vi "TLB Native Dynamic Events ver 0.17c.vi"() -> ()   [LabVIEW 2018]
uses:
  Labview Training Phase 2/Enum Controls/States for Action Engine.ctl
  TLB Type Definitions/State Type Definitions, for 0.26d versions and later.ctl
  TLB Type Definitions/Intruction Type Definitions.ctl
  TLB Type Definitions/Encoder cluster.ctl
  TLB Type Definitions/PING CLUSTER.ctl
  <vilib>/Studica/Studica Toolkit/NavX/NavX.lvlib
  <vilib>/Studica/Studica Toolkit/Background/DIO Channel.ctl
  Underlying VI's/NavX VI/navX type def.ctl
  <vilib>/Studica/Studica Toolkit/Background/I2C Channel.ctl
  TLB Type Definitions/Vision cluster.ctl
  <vilib>/NI_Real-Time Target Support.lvlib
  TLB Type Definitions/Stepper cluster.ctl
  Experimental VI's/Archived VI's/MOTOR CONTROL NO PID Type Def.ctl
  Underlying VI's/I2C Master VI/I2C MASTER Type Def.ctl
  Underlying VI's/I2C Master VI/I2C_MASTER_WRITE_NEW Type Def.ctl
  <vilib>/userdefined/High Color/IMAQdx.ctl
  Underlying VI's/I2C Master VI/Arduino_Interfacing.ctl
  TLB Type Definitions/Yaw Cluster.ctl
  TLB Type Definitions/Time cluster.ctl
  TLB Type Definitions/Y Stepper cluster.ctl
  Underlying VI's/Modified webcam FGV/Webcam AE.ctl
  Underlying VI's/Elasped Timer/Elapsed timer control.ctl
  Underlying VI's/Motor Control VI with PID/MOTOR CONTROL WITH PID AE DATA MODE TYPE DEF.ctl
  Underlying VI's/Motor Control VI with PID/MOTOR CONTROL WITH PID AE DIRECTION TYPE DEF.ctl
  TLB Type Definitions/IR Sensor Type Def.ctl
  <vilib>/myRIO/Common/Instrument Driver Framework/myRIO v1.0/AI/typedefs/AI Channels Enum.ctl
  <vilib>/myRIO/Common/Instrument Driver Framework/myRIO v1.0/AI/typedefs/AI Channels List.ctl
  <vilib>/Utility/RT CPU Load.ctl
panel:
  out "Left IR Sensor":dbl
  out "Obstacle detected":bool
  out "Speed & distance":T1
  out "Object Center Coordinates":cluster{"x":sgl, "y":sgl}
  out "Object detection cluster":T2
  out "Time up flag":bool
  out "Task selection":u8
  in  "Object recognition mode":enum16{"Ball", "Soap", "Gel", "Pipe", "None"}(ring)
  out "NavX Readings":T3
  out "Arduino Data":T4
  out "CPU loads":T5[](array[typedef]) {"ISR (%)" format="%#.2f"; "Idle (%)" format="%#.2f"; "Background (%)" format="%#.2f"; "Normal (%)" format="%#.2f"; "Above Normal (%)" format="%#.2f"; "High (%)" format="%#.2g"; "Timed Structures (%)" format="%#.2g"; "Time Critical (%)" format="%#.2g"; "Total (%)" format="%#.2g"}
  out "TASK ENABLE":bool
  out "Rising Edge":bool
  in  "Green LED":bool
  out "I2C Error":errorcluster
  out "State Logic":T6=enum."Startup"
  out "elements":T7[](array[typedef])
  in  "STOP TASK":bool
  in  "OK Button":bool
  in  "STOP":bool
  out "error out":errorcluster
  out "Action Queue Items":i32
  out "State Logic Queue Items":i32
  out "Action Queues items":string[](array[string])=["Hardware reset", "Software reset", ""]
  out "Action State":string
  # "System Health Status Update"
  # "VISION"
  # "TLB FRAMEWORK STATUS"
  # "Test Programme written by Calvin Loke    Dated: 28 Aug 2019\nTest Programme revised by Dr Alex See   Dated 30 Aug 2019\n\nRevision date: 20/03/2020\nProgramme version:   TLB Native Dynamic Events ver 0.14a"
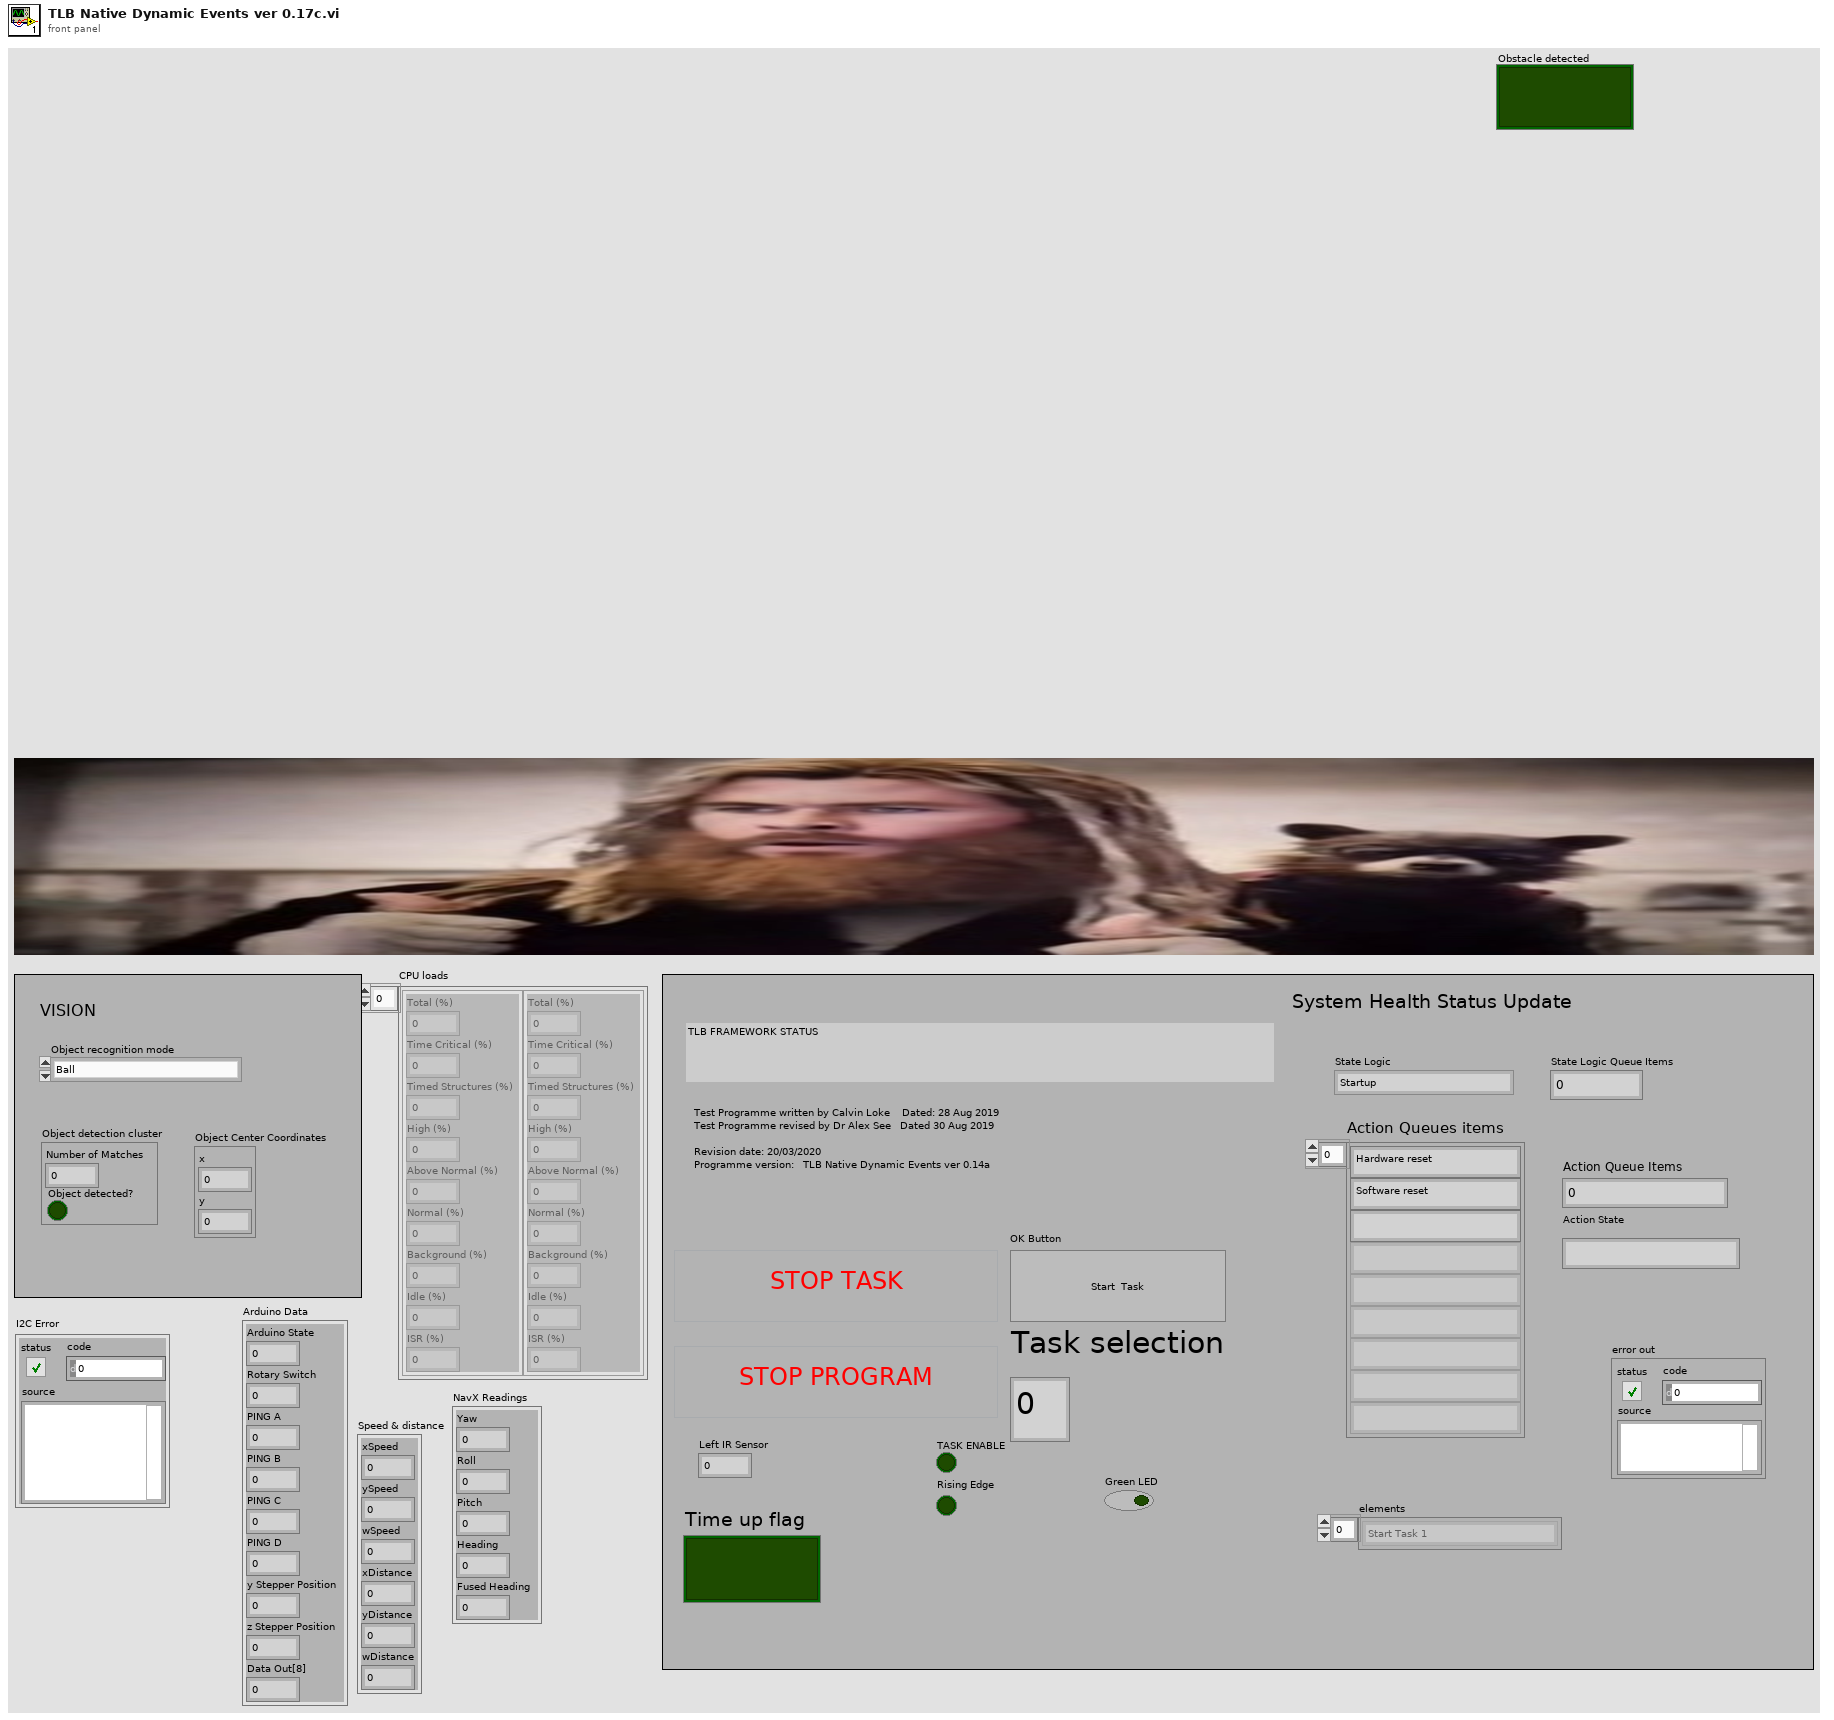
[diagram p1: front panel]
types:
  T1 = cluster{"xSpeed":dbl, "ySpeed":dbl, "wSpeed":dbl, "xDistance":dbl, "yDistance":dbl, "wDistance":dbl}
  T2 = cluster{"Number of Matches":i32, "Object detected?":bool}
  T3 = cluster{"Yaw":dbl, "Roll":dbl, "Pitch":dbl, "Heading":dbl, "Fused Heading":dbl}
  T4 = cluster{"Arduino State":u8, "Rotary Switch":u8, "PING A":u8, "PING B":u8, "PING C":u8, "PING D":u8, "y Stepper Position":u8, "z Stepper Position":u8, "Data Out[8]":u8}
  T5 = typedef "NI_Real-Time Target Support.lvlib/RT CPU Load.ctl" = cluster{"Total (%)":dbl, "Time Critical (%)":dbl, "Timed Structures (%)":dbl, "High (%)":dbl, "Above Normal (%)":dbl, "Normal (%)":dbl, "Background (%)":dbl, "Idle (%)":dbl, "ISR (%)":dbl}
  T6 = typedef "State Type Definitions.ctl" = enum16{"None", "Startup", "Move to Angle", "True Stop", "Idle", "Shutdown", "Task 1A", "Task 1B", "Task 2:Raise Arm", "Task 2:Sensor Mode", "Task 2:Reverse Mode", "Task 3", "Task 4_A", "Task 4_B", "Task 4_C", "Task 4_D", "Task 5A", "Task 5B", "Task 5C", "Task 5D", "Task 5E: POSITION ARM", "Task 5F: ARM GRAB HEIGHT", "Task 5G: CLOSE CLAW", "Task 5H: RAISE ARM", "Task 6_A", "Task 6_B", "Task 7", "Task 8A: RAISE ARM", "Task 8B: MOVE TO BOX", "Task 8C: CAM BURST", "Task 8D: PROCESS IMAGE", "Task 8E: ROBOT ADJUST", "Task 8F: CAM BURST 2", "Task 8G: PROCESS IMAGE 2", "Task 8H: ARM ADJUST", "Task 8I: ARM GRAB HEIGHT", "Task 8J: CLOSE CLAW", "Task 8K: RAISE MY SWORD", "Task 9A: Raise Arm", "Task 9B: Rotate to Angle", "Task 9C: Detect Box", "Task 9D: MOVE FORWARD", "Task 9E: MOVE LEFT", "Task 9F: SCAN IMAGE", "Task 9G: PROCESS COLOUR", "Task 9H: MOVE RIGHT", "Task 9I: SCAN IMAGE", "Task 9J: PROCESS COLOUR", "Task 9K: ROTATE 90 CW", "Task 9L: MOVE FORWARD", "Task 9M: MOVE RIGHT", "Task 9N: SCAN IMAGE", "Task 9O: PROCESS COLOUR", "Task 9P: MOVE RIGHT", "Task 9Q: SCAN IMAGE", "Task 9R: PROCESS COLOUR", "Task A1: Raise Arm", "Task A2: Rotate to Angle", "Task A3: Move Forward", "Task A4: Rotate CW 90"}
  T7 = typedef "Intruction Type Definitions.ctl" = enum16{"None", "Start Task 1", "Start Task 2", "Start Task 3", "Start Task 4", "Start Task 5", "Start Task 6", "Start Task 7", "Start Task 8 - BALL", "Start Task 8 - Gel", "Start Task 8 - Pipe", "Start Task 8 - Soap", "Start Task 9", "Start Task A", "Start Task B", "Exit"}
  T8 = typedef "IR Sensor Type Def.ctl" = cluster{"Left IR Sensor":dbl, "Arm IR Sensor":dbl, "Bottom IR Sensor":dbl}
  T9 = typedef "Y Stepper cluster.ctl" = cluster{"yStepper desired":u8}
  T10 = typedef "Time cluster.ctl" = cluster{"Time up flag":bool, "SET TIME TO CHECK":dbl}
  T11 = typedef "Yaw Cluster.ctl" = cluster{"Yaw":dbl, "Compass":dbl}
  T12 = typedef "Stepper cluster.ctl" = cluster{"y Stepper Position":u8, "z Stepper Position":u8}
  T13 = typedef "DIO Channel.ctl" = enum16{"Not Connected", "A/DIO1", "A/DIO2", "A/DIO3", "A/DIO4", "A/DIO5", "A/DIO6", "A/DIO7", "A/DIO13", "B/DIO1", "B/DIO2", "B/DIO3", "B/DIO4", "B/DIO5", "B/DIO6", "B/DIO7", "B/DIO13", "C/DIO0", "C/DIO1", "C/DIO2", "C/DIO3", "C/DIO4", "C/DIO5", "C/DIO6", "C/DIO7"}
  T14 = typedef "Vision cluster.ctl" = cluster{"Recognized Object":bool, "Object X coordinate":dbl, "Object Y coordinate":dbl}
  T15 = typedef "PING CLUSTER.ctl" = cluster{"PING_A":u8, "PING_B":u8, "PING_C":u8, "PING_D":u8}
  T16 = typedef "Encoder cluster.ctl" = cluster{"xDistance":dbl, "yDistance":dbl, "wDistance":dbl}
  T17 = cluster{"DIO Channel":T13, "FPGA VI Reference Out":refnum<k20>}
  T18 = typedef "navX type def.ctl" = enum16{"Get i2C reference", "Read Values", "Zero Yaw"}
  T19 = typedef "Arduino_Interfacing.ctl" = enum16{"Initialize", "Write to Arduino", "Read From Arduino"}
  T20 = typedef "I2C Channel.ctl" = enum16{"Not Connected", "A", "B"}
  T21 = typedef "States for Action Engine.ctl" = enum16{"Initialize", "Write", "Read"}
  T22 = cluster{"I2C Ref Out":cluster{"I2C Channel":T20, "FPGA VI Reference Out":refnum<k20>}, "Connected":bool, "Slave Address (7-bit)":u8, "Registry":u8[]}
  T23 = typedef "IMAQ Image.ctl" = refnum<image>
  T24 = typedef "State Type Definitions.ctl" = enum16{"None", "Startup", "Move to Angle", "True Stop", "Idle", "Shutdown", "Task 1", "Task 2:Raise Arm", "Task 2:Sensor Mode", "Task 2:Reverse Mode", "Task 3", "Task 4_A", "Task 4_B", "Task 4_C", "Task 4_D", "Task 5A: ARM CAM HEIGHT", "Task 5B: MOVE TO BOX", "Task 5C: CAM BURST", "Task 5D: PROCESS IMAGE", "Task 5E: POSITION ARM", "Task 5F: ARM GRAB HEIGHT", "Task 5G: CLOSE CLAW", "Task 5H: RAISE ARM", "Task 5_F", "Task 5G", "Task 5H", "Task 5I", "Task 6_A", "Task 6_B", "Task 7", "Task 8", "Task 9A: Raise Arm", "Task 9B: Rotate to Angle", "Task 9C: Rotation alignmnet", "Task B"}
  T25 = typedef "MOTOR CONTROL WITH PID AE DIRECTION TYPE DEF.ctl" = enum16{"y-axis movement", "x-axis movement", "rotation", "stop", "reset encoders"}
  T26 = typedef "MOTOR CONTROL WITH PID AE DATA MODE TYPE DEF.ctl" = enum16{"Init AE", "Write to AE", "Read from AE"}
  T27 = typedef "Elapsed timer control.ctl" = enum16{"Start", "Pause", "Initialize"}
  T28 = typedef "I2C_MASTER_WRITE_NEW Type Def.ctl" = enum16{"Ultrasonic sensors", "Stepper origin", "zStepper 13.3k", "zStepper 13k", "zStepper 12k", "zStepper 11k", "zStepper 10k", "zStepper 9k", "zStepper 8k", "zStepper 7k", "zStepper 6k", "zStepper 5k", "zStepper 4k", "zStepper 3k", "zStepper 2k", "zStepper 1k", "zStepper 900", "zStepper 800", "zStepper 700", "zStepper 600", "zStepper 500", "zStepper 400", "zStepper 300", "zStepper 200", "zStepper 100", "zStepper 0", "yStepper control", "Open Claw", "Close Claw", "Soft Reset"}
  T29 = typedef "Webcam AE.ctl" = enum16{"Initialize Camera", "Open Camera", "Continuous Acquisition", "Close Camera", "Retrieve Image", "Dispose Camera Image Buffer"}
  T30 = typedef "IMAQdx.ctl" = refnum<k21>
  T31 = typedef "Webcam AE.ctl" = enum16{"Initialize Camera", "Open Camera", "Continuous Acquisition", "Close Camera", "Retrieve Image", "Dispose Image Buffers"}
  T32 = typedef "MOTOR CONTROL NO PID Type Def.ctl" = enum16{"Init", "Front Back", "Left Right", "Rotate", "Stop", "Latch"}
  T33 = typedef "AI Channels List.ctl" = T34[]
  T34 = typedef "AI Channels Enum.ctl" = enum16{"Not Connected", "AudioIn/Left", "AudioIn/Right", "C/AI0", "C/AI1", "A/AI0", "A/AI1", "A/AI2", "A/AI3", "A/AI4", "A/AI5", "A/AI6", "A/AI7", "B/AI0", "B/AI1", "B/AI2", "B/AI3", "B/AI4", "B/AI5", "B/AI6", "B/AI7", "AI/AI0", "AI/AI1", "AI/AI2", "AI/AI3", "A/AI0 (DIFF)", "A/AI1 (DIFF)", "A/AI2 (DIFF)", "A/AI3 (DIFF)", "B/AI0 (DIFF)", "B/AI1 (DIFF)", "B/AI2 (DIFF)", "B/AI3 (DIFF)"}
  T35 = typedef "I2C MASTER Type Def.ctl" = enum16{"Last State", "Mode 0", "Mode 1", "Mode 2", "Mode 3", "Mode 4", "Mode 5", "Mode 6", "Mode 7", "Mode 8", "Mode 9", "Mode 10"}
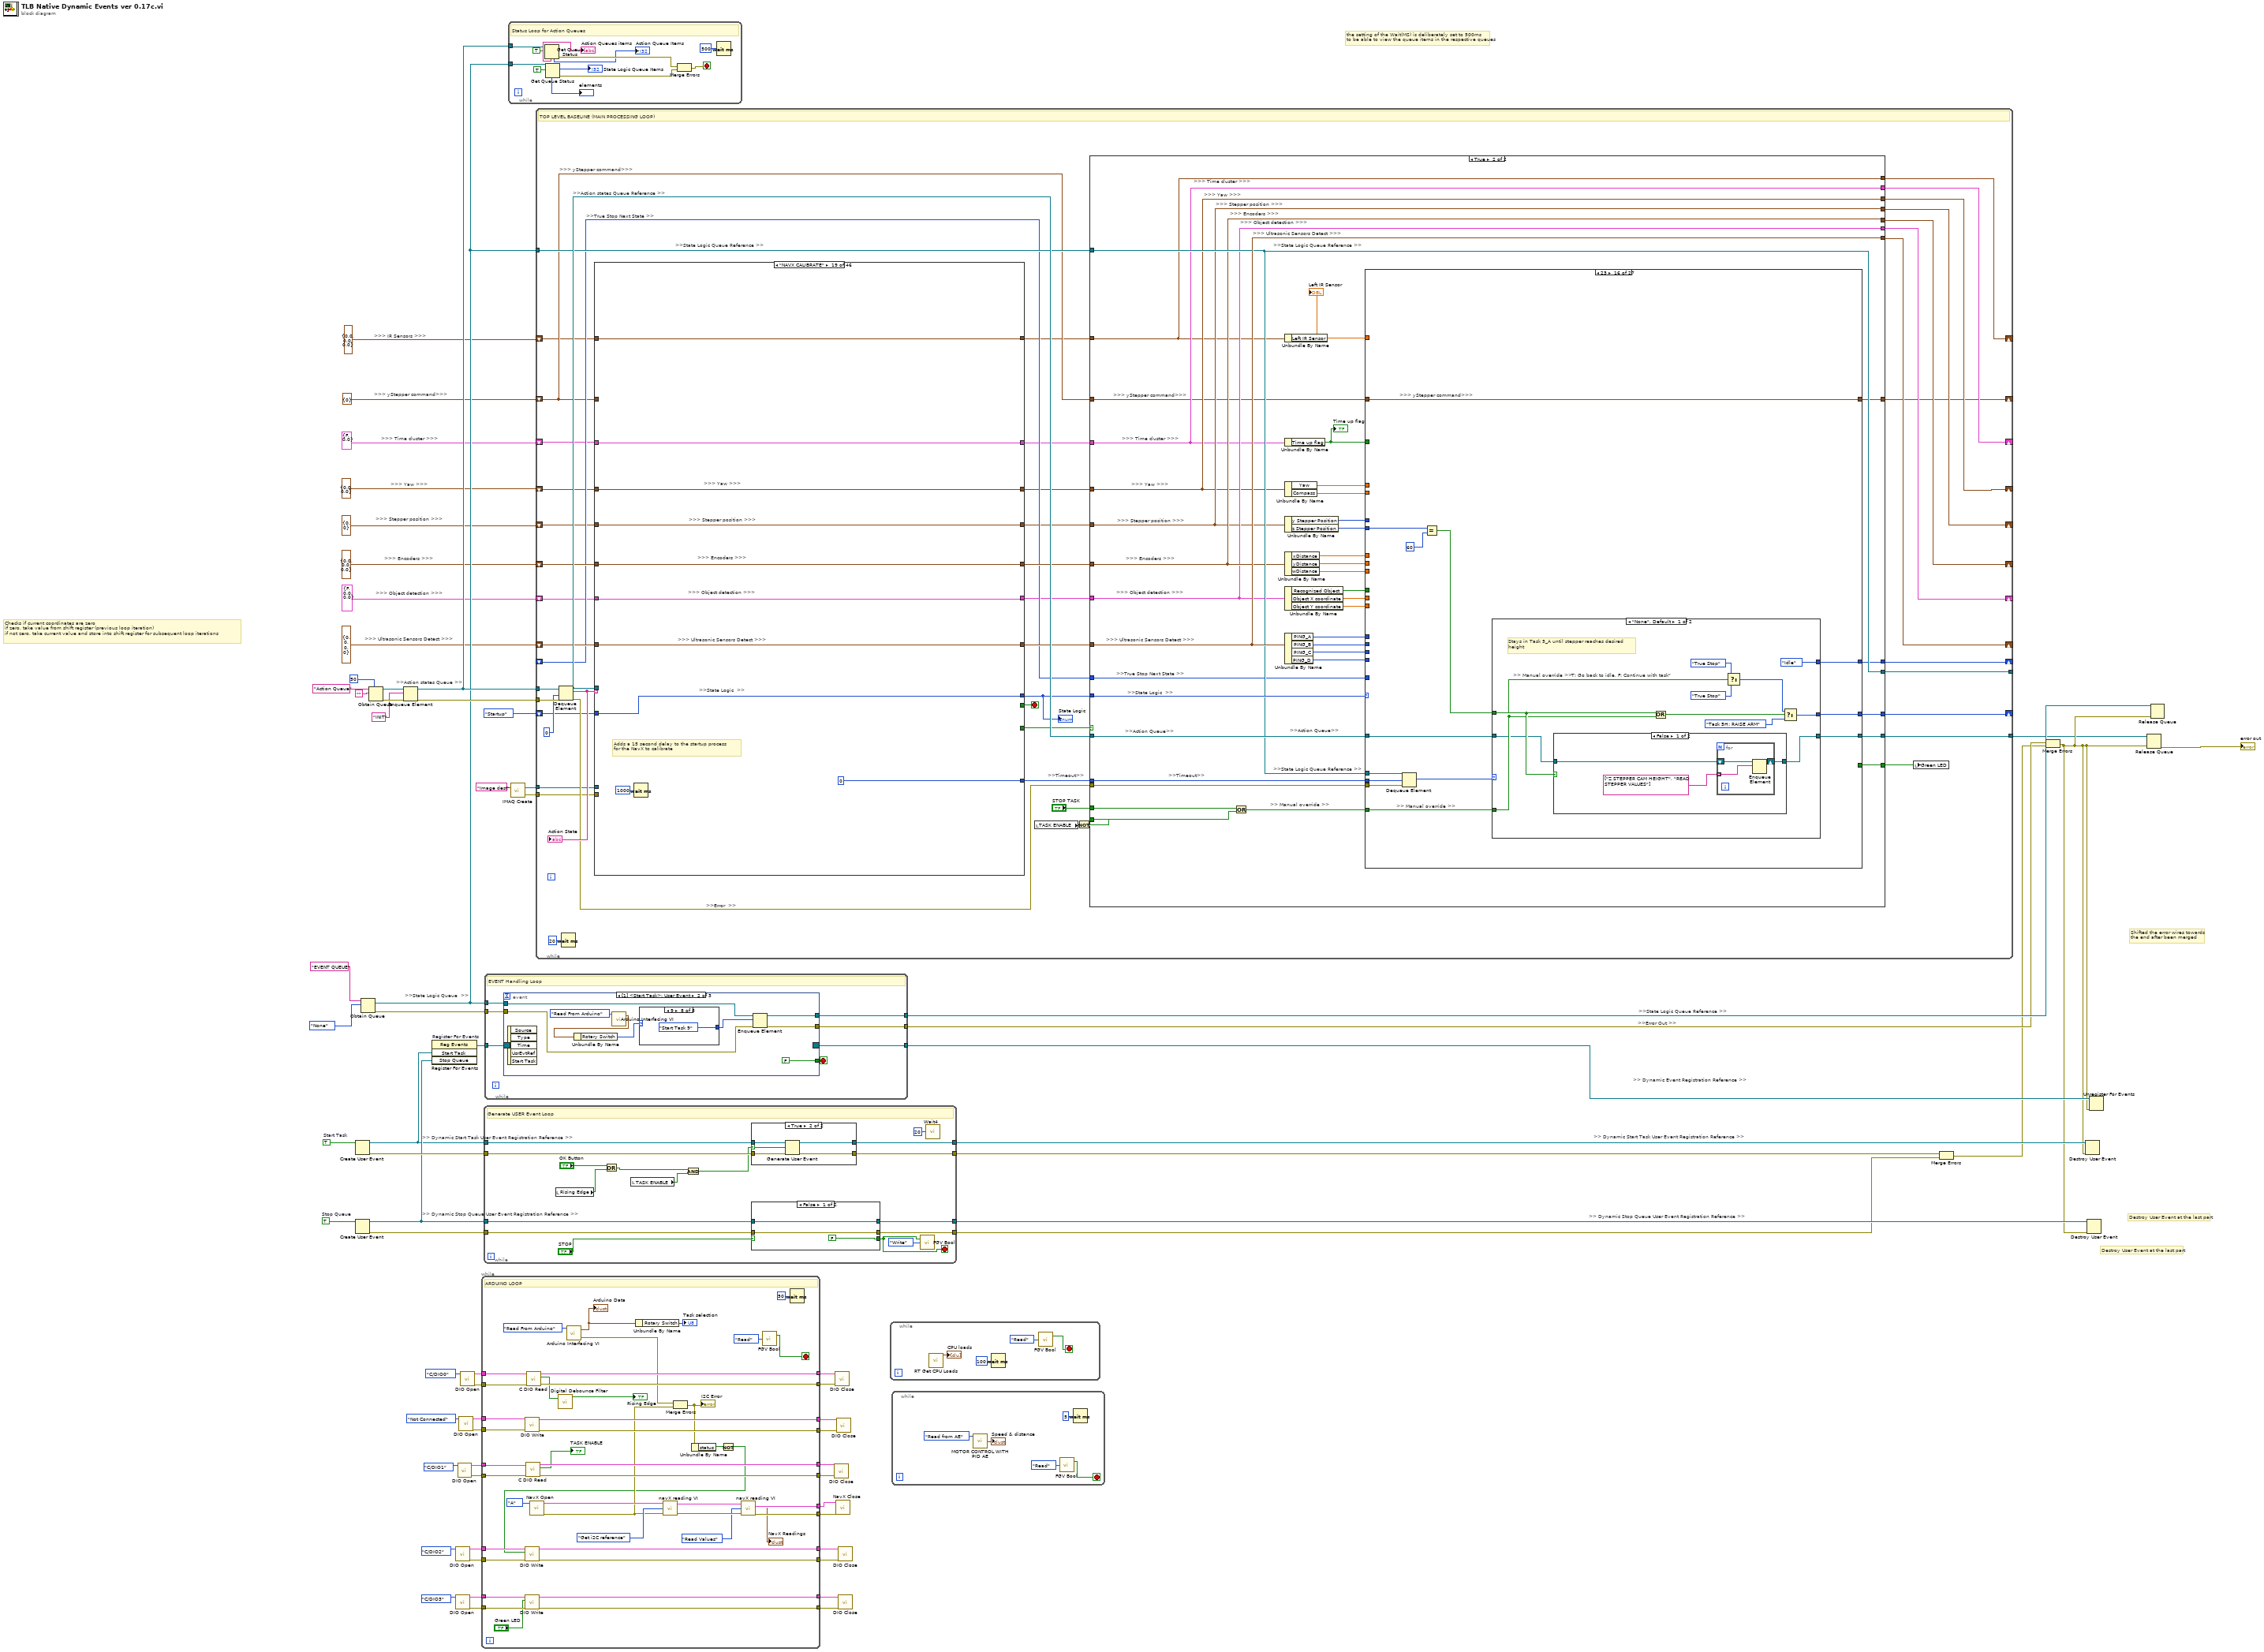
[diagram p0: block diagram]
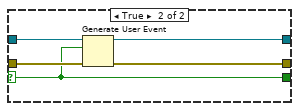
[diagram p2: hidden frame]
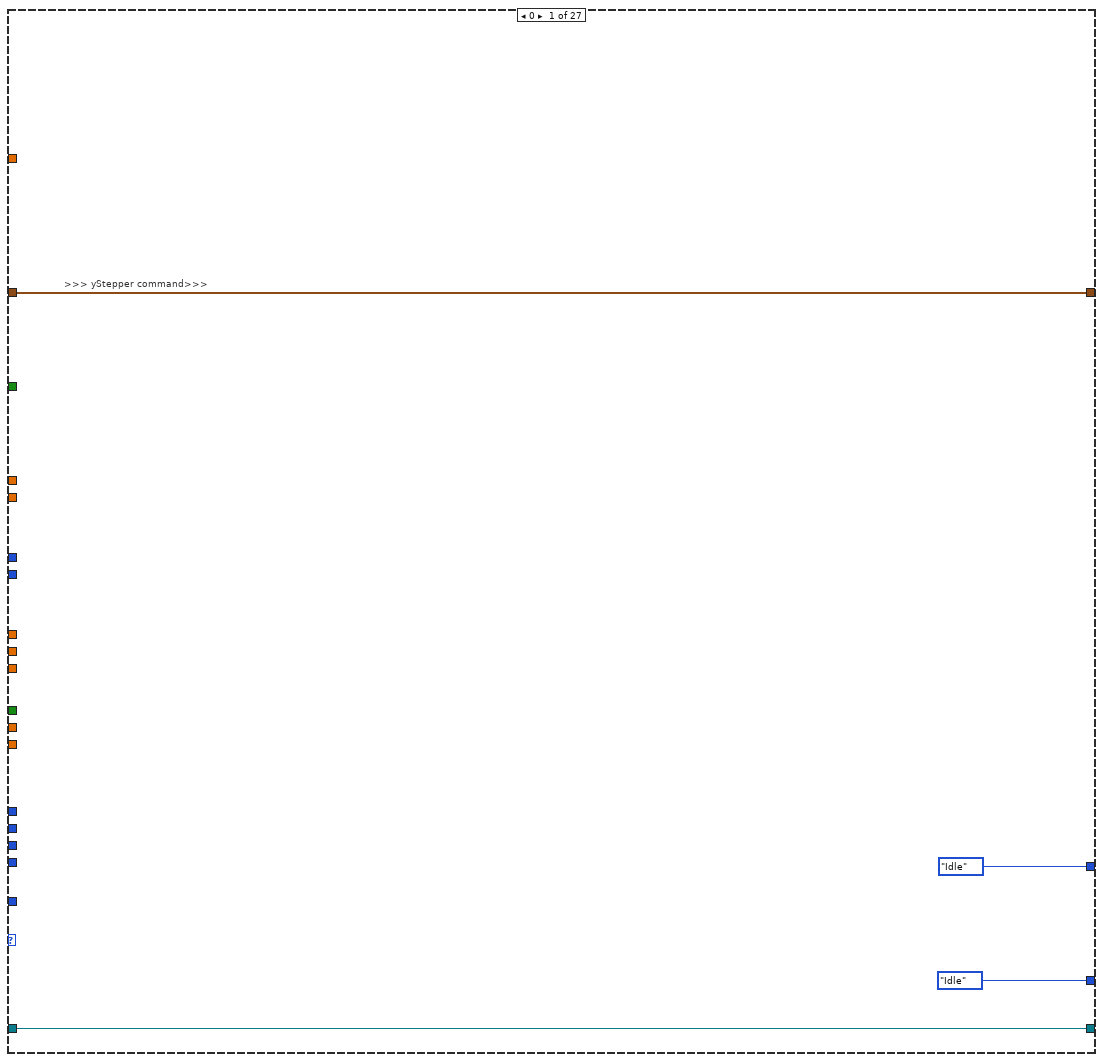
[diagram p5: hidden frame]
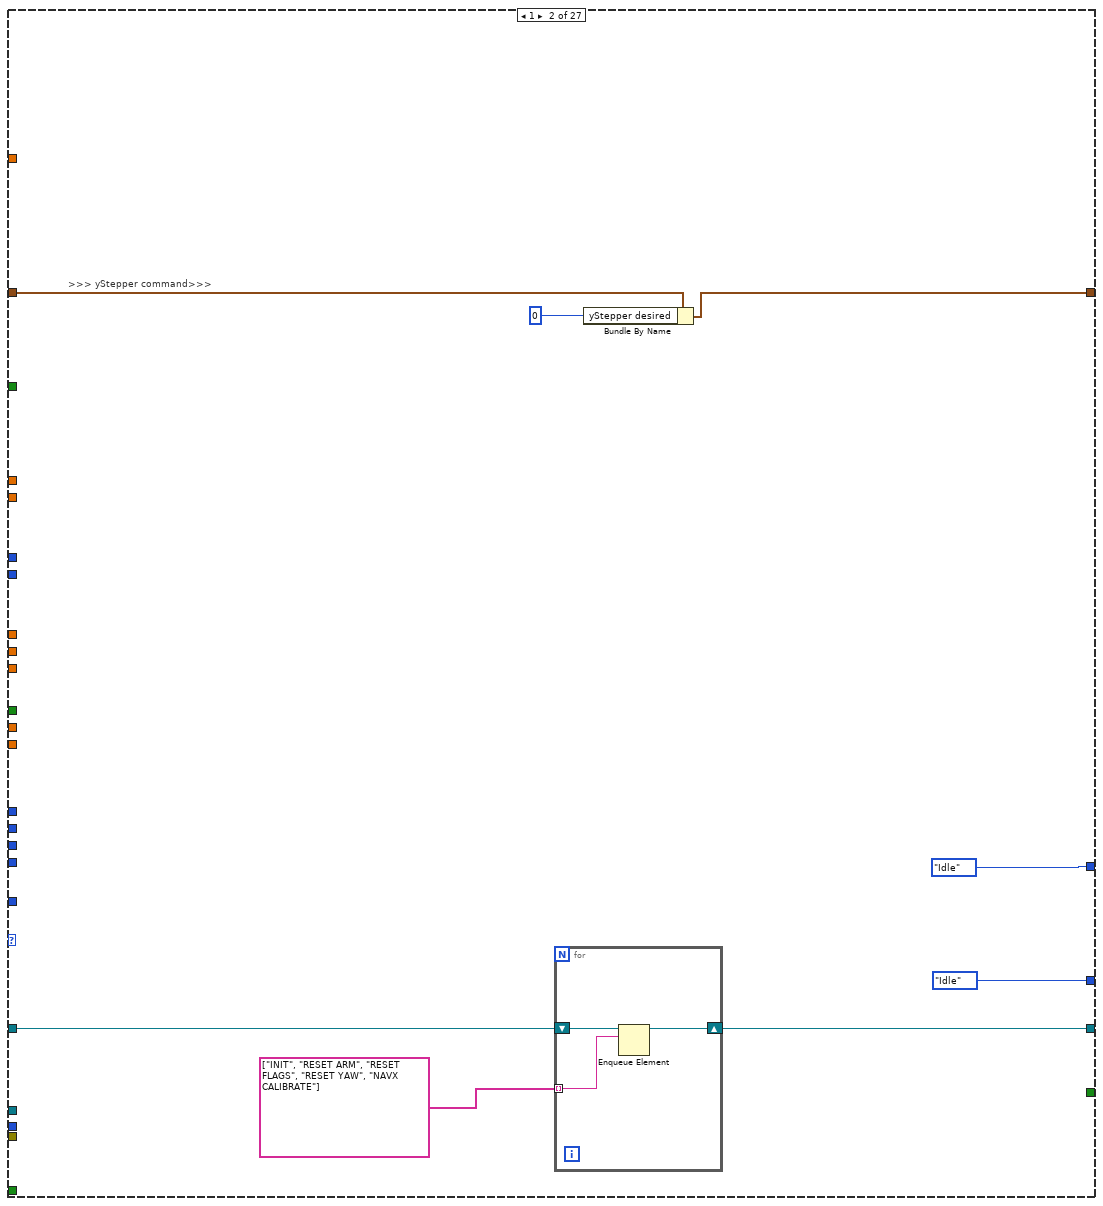
[diagram p6: hidden frame]
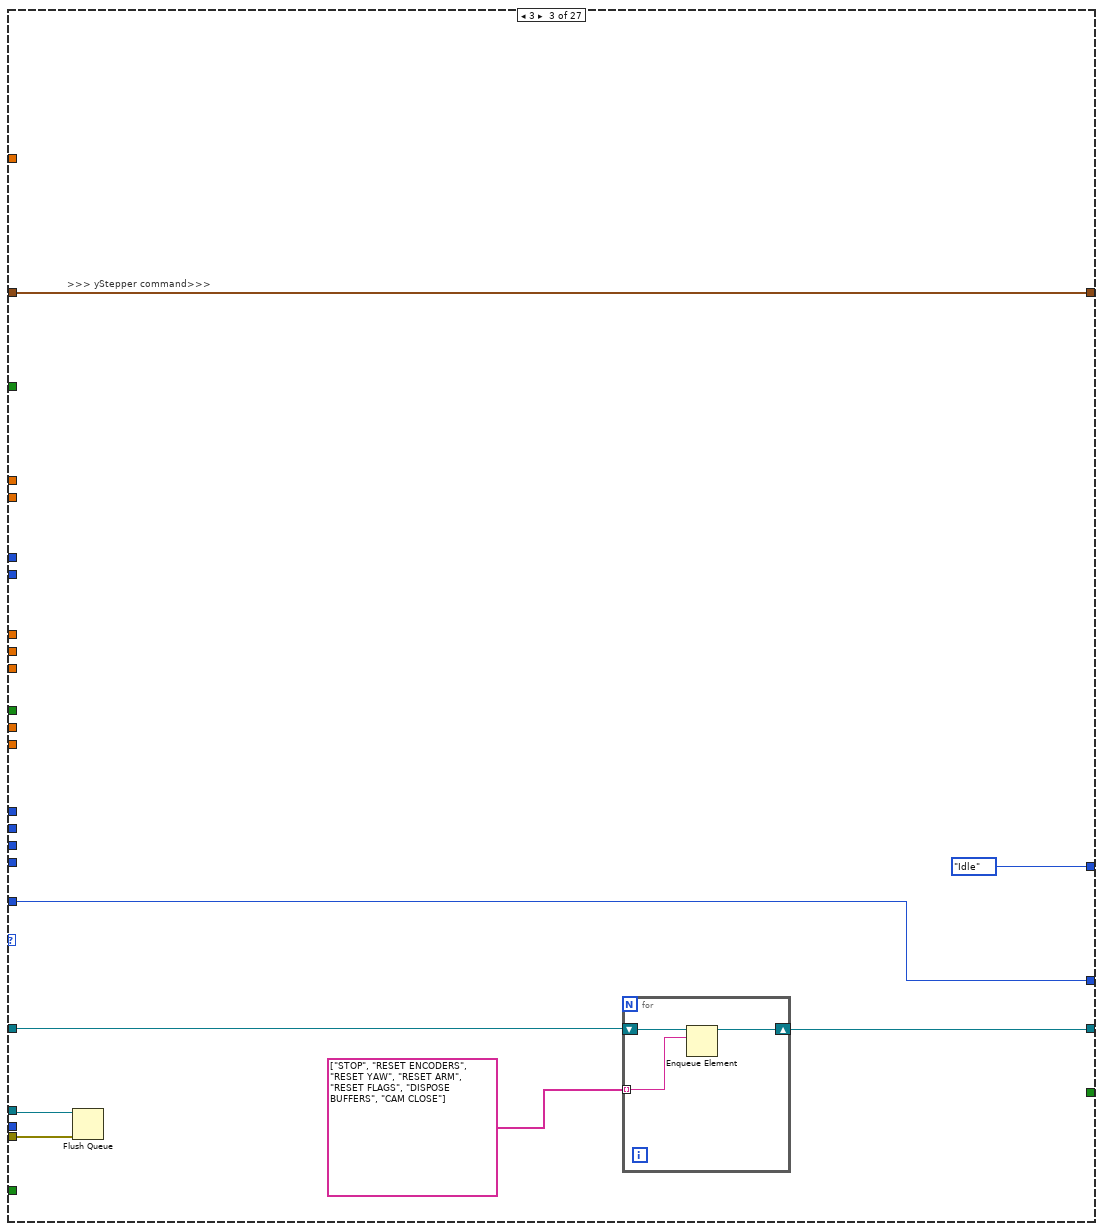
[diagram p7: hidden frame]
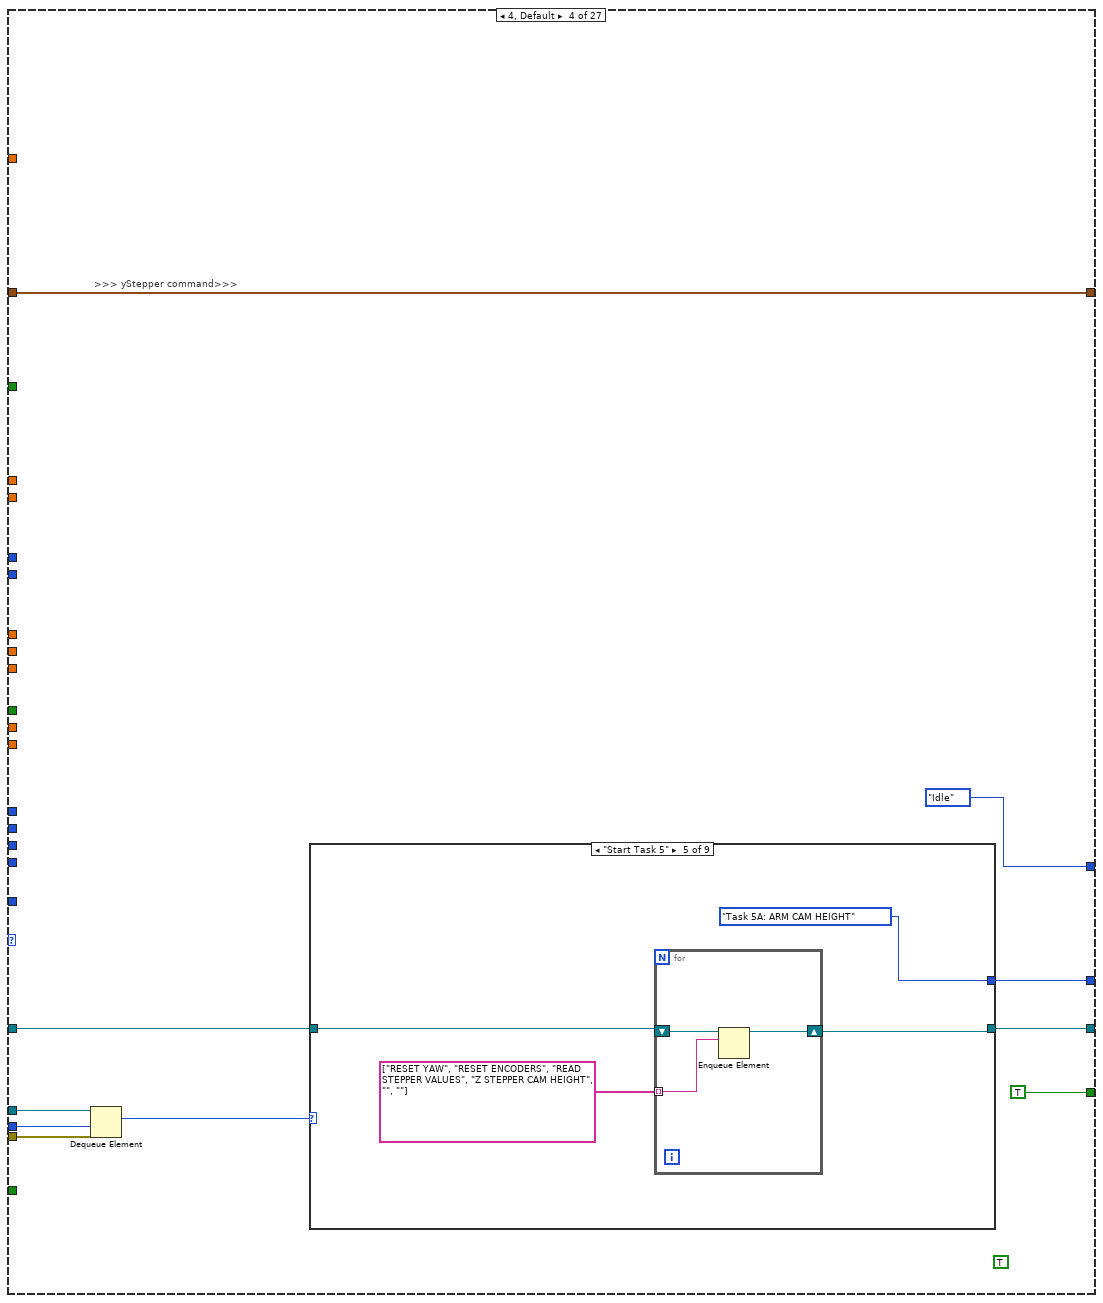
[diagram p8: hidden frame]
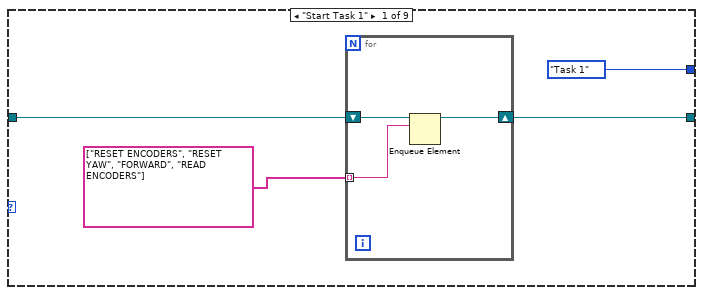
[diagram p9: hidden frame]
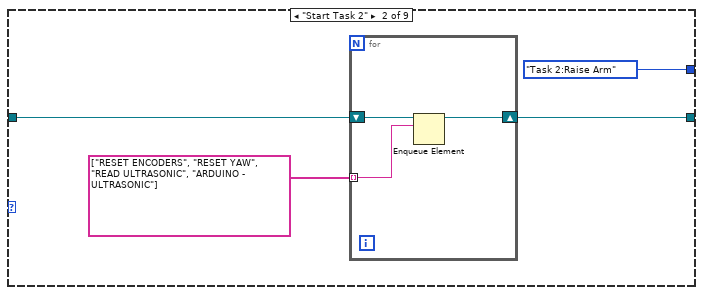
[diagram p10: hidden frame]
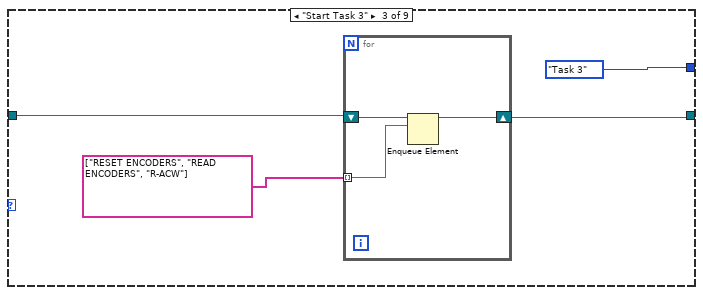
[diagram p11: hidden frame]
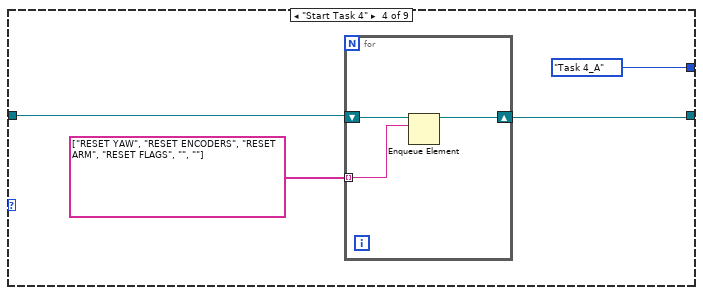
[diagram p12: hidden frame]
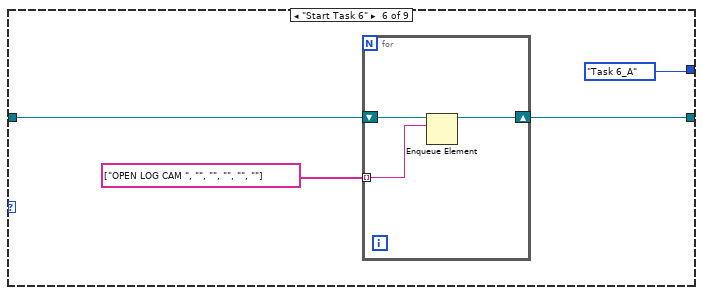
[diagram p13: hidden frame]
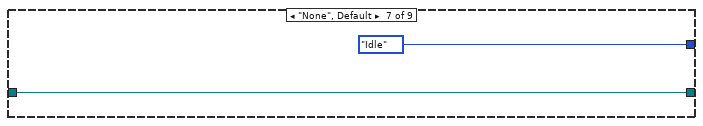
[diagram p14: hidden frame]
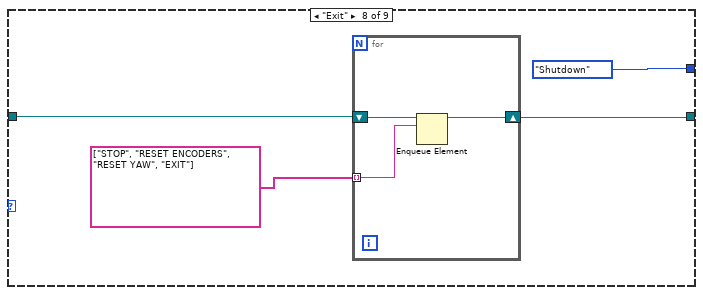
[diagram p15: hidden frame]
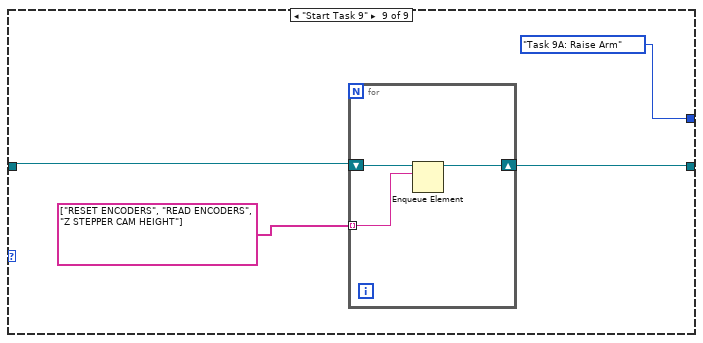
[diagram p16: hidden frame]
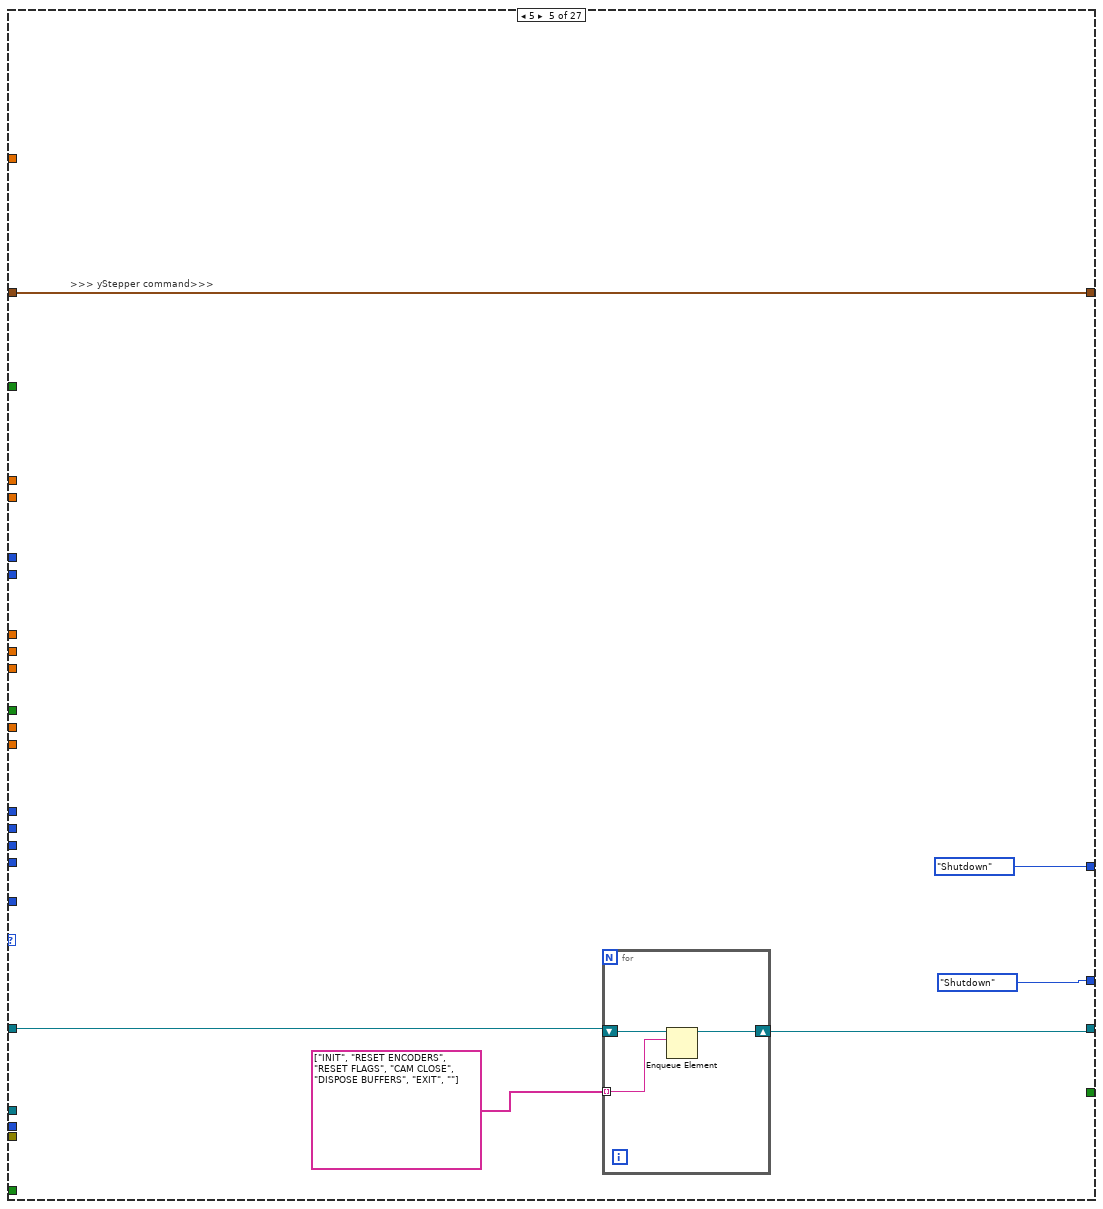
[diagram p17: hidden frame]
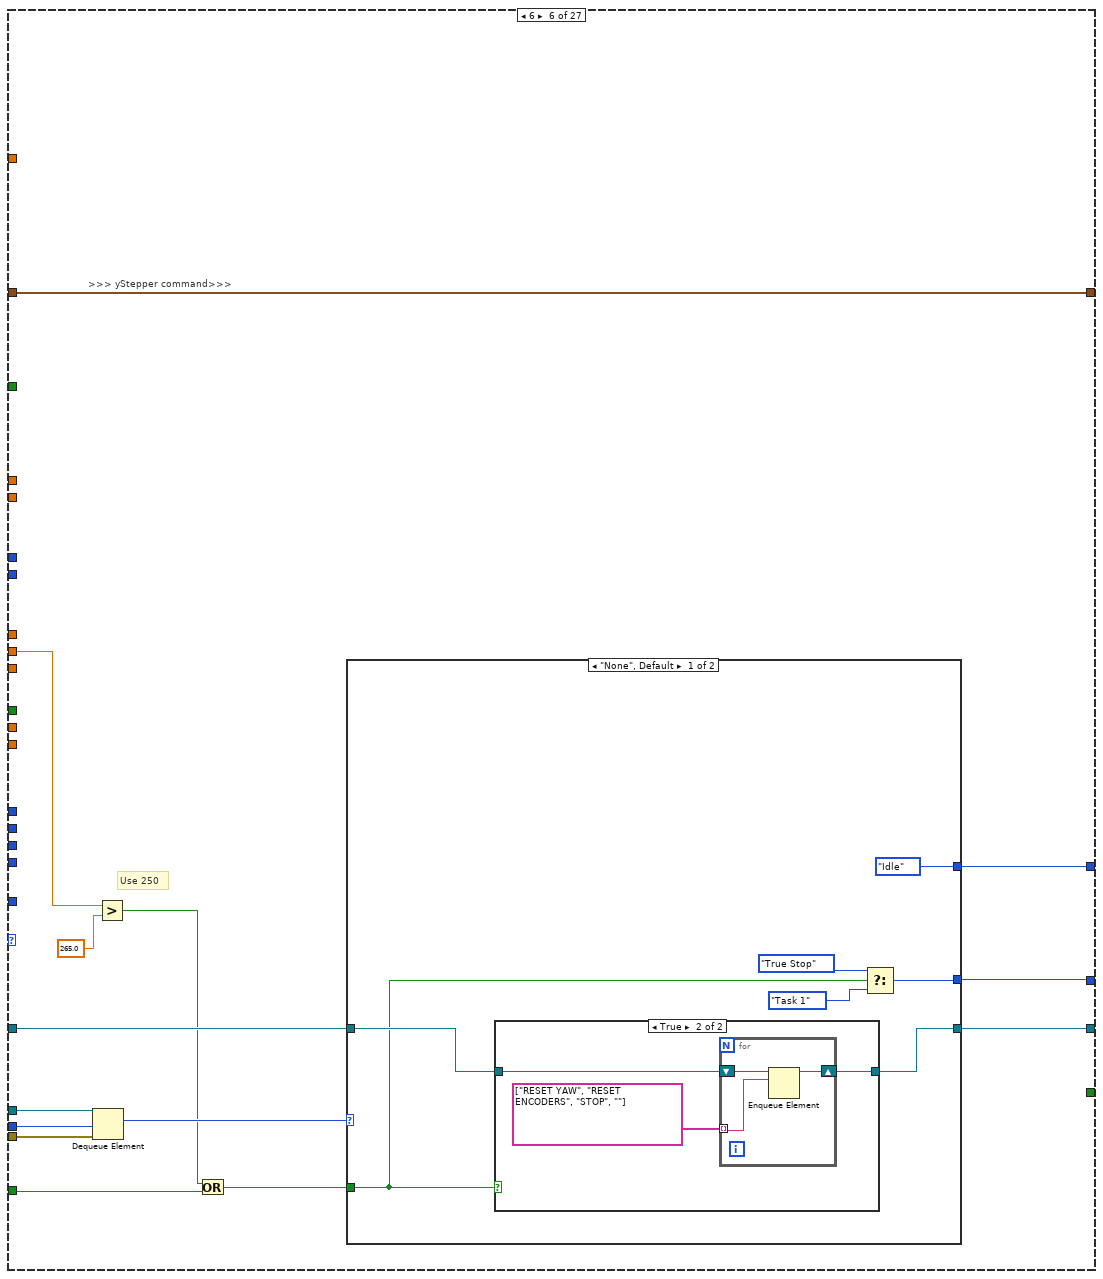
[diagram p18: hidden frame]
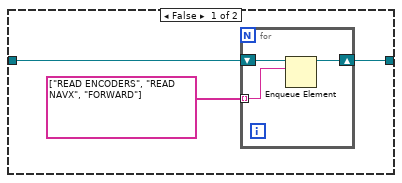
[diagram p19: hidden frame]
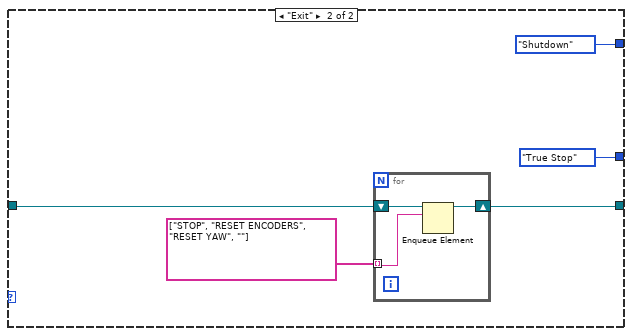
[diagram p20: hidden frame]
diagram:
  w69 = TRUE  # Stop Queue
  w68 = TRUE  # Start Task
  # ">>> IR Sensors >>>"
  # "Checks if current coordinates are zero\nif zero, take value from shift register (previous loop iteration)\nif not zero, take current value and store into shift register for subsequent loop iterations"
  # ">>> yStepper command>>>"
  # ">>> Time cluster >>>"
  # ">>> Yaw >>>"
  # ">>> Stepper position >>>"
  # ">>> Encoders >>>"
  # ">>> Object detection >>>"
  # ">>> Ultrasonic Sensors Detect >>>"
  # "the setting of the Wait(MS) is deliberately set to 500ms\nto be able to view the queue items in the respective queues"
  # ">>Error Out >>"
  # ">> Dynamic Stop Queue User Event Registration Reference >>"
  # ">> Dynamic Start Task User Event Registration Reference >>"
  # ">> Dynamic Stop Queue User Event Registration Reference >>"
  # ">> Dynamic Start Task User Event Registration Reference >>"
  # ">> Dynamic Event Registration Reference >>"
  # ">>Action states Queue >>"
  # ">>State Logic Queue  >>"
  # ">>State Logic Queue Reference >>"
  # "Destroy User Event at the last part"
  # "Destroy User Event at the last part"
  # "Shifted the error wires towards\nthe end after been merged"
  n1 = Create User Event(user event datatype=w68) -> (user event=w60:refnum<user-event>, error out=w65:errorcluster)  [unwired: 1 in]
  n2 = Create User Event(user event datatype=w69) -> (user event=w61:refnum<user-event>, error out=w64:errorcluster)  [unwired: 1 in]
  n3 = Obtain Queue(name (unnamed)="EVENT QUEUE", element data type=Intruction_Type_Definitions."None" ("Enum")) -> (queue out=w46:refnum<queue>, error out=w52:errorcluster)  [unwired: 3 in, 1 out]
  n4 = Obtain Queue(max queue size (-1, unlimited)=50, name (unnamed)="Action Queue", element data type="") -> (queue out=w55:refnum<queue>, error out=w51:errorcluster)  [unwired: 2 in, 1 out]
  n5 = Enqueue Element(queue=w55, element="INIT", error in (no error)=w51) -> (queue out=w47:refnum<queue>, error out=w50:errorcluster)  [unwired: 1 in, 1 out]
  n6 = register-events "Register For Events"(w60, w61) -> (reference out=w59:refnum<event-registration>)  [unwired: 2 in, 1 out]
  n7 = call <vilib>:"DIO Open.vi"("DIO Channel"=DIO_Channel."C/DIO2") -> ("error out"=w16:errorcluster, "DIO Info Out"=w17:T17)  [unwired: 9 in]
  n8 = call <vilib>:"DIO Open.vi"("DIO Channel"=DIO_Channel."C/DIO3") -> ("error out"=w11:errorcluster, "DIO Info Out"=w12:T17)  [unwired: 9 in]
  n9 = call <vilib>:"DIO Open.vi"("DIO Channel"=DIO_Channel."C/DIO1") -> ("error out"=w24:errorcluster, "DIO Info Out"=w25:T17)  [unwired: 9 in]
  n10 = call <vilib>:"DIO Open.vi"("DIO Channel"=DIO_Channel."Not Connected") -> ("error out"=w29:errorcluster, "DIO Info Out"=w31:T17)  [unwired: 9 in]
  n11 = call <vilib>:"DIO Open.vi"("DIO Channel"=DIO_Channel."C/DIO0") -> ("error out"=w34:errorcluster, "DIO Info Out"=w37:T17)  [unwired: 9 in]
  n12 = while {
    tunnel: w37 -> [w110]
    tunnel: [w109] -> w35
    tunnel: w34 -> [w108]
    tunnel: [w107] -> w33
    tunnel: w31 -> [w104]
    tunnel: [w103] -> w30
    tunnel: w29 -> [w102]
    tunnel: [w101] -> w28
    tunnel: [w100] -> w26
    tunnel: w25 -> [w99]
    tunnel: w24 -> [w98]
    tunnel: [w97] -> w23
    tunnel: w17 -> [w91]
    tunnel: w16 -> [w90]
    tunnel: [w89] -> w15
    tunnel: [w88] -> w14
    tunnel: w12 -> [w87]
    tunnel: w11 -> [w86]
    tunnel: [w85] -> w10
    tunnel: [w84] -> w9
    tunnel: [w78] -> w6
    tunnel: [w77] -> w7
    stop <- w112 stop-if-true
    # "ARDUINO LOOP"
    n13 = call <vilib>:"DIO Write.vi"("error in (no error)"=w86, "Input"="Green LED", "DIO Info In"=w87) -> ("error out"=w84:errorcluster, "DIO Info Out"=w85:T17)  [unwired: 7 in]
    n14 = call <vilib>:"DIO Write.vi"("error in (no error)"=w102, "DIO Info In"=w104) -> ("error out"=w101:errorcluster, "DIO Info Out"=w103:T17)  [unwired: 8 in]
    n15 = call <vilib>:"C DIO Read.vi"("error in (no error)"=w98, "DIO Info In in"=w99) -> ("error out"=w97:errorcluster, "IN"=→"TASK ENABLE":bool, "DIO Info In out"=w100:T17)  [unwired: 7 in]
    n16 = call <vilib>:"C DIO Read.vi"("error in (no error)"=w108, "DIO Info In in"=w110) -> ("error out"=w107:errorcluster, "IN"=w106:bool, "DIO Info In out"=w109:T17)  [unwired: 7 in]
    n17 = call <vilib>:"NavX Open.vi"("I2C Channel"=I2C_Channel."A") -> ("error out"=w93:errorcluster, "NavX Info"=w95:T22)  [unwired: 9 in]
    n18 = call "Digital Debounce Filter.vi"("Boolean input"=w106) -> ("Rising Edge"=→"Rising Edge":bool)  [unwired: 1 in, 2 out]
    n19 = call "Arduino Interfacing VI.vi"("AE Mode"=Arduino_Interfacing."Read From Arduino") -> ("error out"=w81:errorcluster, "Arduino Data"=w74:T4)  [unwired: 3 in]
    "Arduino Data" <- w74
    n20 = Unbundle By Name(w74) -> ("Rotary Switch"=→"Task selection":u8)
    n21 = call "navX reading VI.vi"("NavX Info In"=w95, "Mode"=navX_type_def."Get i2C reference", "error in (no error)"=w93) -> ("NavX Info Out"=w80:T22, "Error Out"=w79:errorcluster)  [unwired: 2 out]
    n22 = Merge Errors(w81, w93) -> (w72:errorcluster)
    "I2C Error" <- w72
    n23 = Unbundle By Name(w72) -> ("status"=w71:bool)
    n24 = Not(x=w71) -> (.not. x?=w70:bool)
    n25 = call <vilib>:"DIO Write.vi"("error in (no error)"=w90, "Input"=w70, "DIO Info In"=w91) -> ("error out"=w88:errorcluster, "DIO Info Out"=w89:T17)  [unwired: 7 in]
    n26 = call "navX reading VI.vi"("NavX Info In"=w80, "Mode"=navX_type_def."Read Values", "error in (no error)"=w79) -> ("NavX Info Out"=w78:T22, "NavX Readings"=→"NavX Readings":T3, "Error Out"=w77:errorcluster)  [unwired: 1 out]
    n27 = call "FGV Bool.vi"("Init/Read/Write State"=States_for_Action_Engine."Read") -> ("Output node"=w112:bool)  [unwired: 2 in, 1 out]
    n28 = Wait (ms)(milliseconds to wait=u32 50) -> ()  [unwired: 1 out]
  }
  n29 = while {
    tunnel: w60 -> [w130]
    tunnel: w61 -> [w129]
    tunnel: [w128] -> w67
    tunnel: [w127] -> w66
    tunnel: w65 -> [w126]
    tunnel: [w125] -> w63
    tunnel: w64 -> [w124]
    tunnel: [w123] -> w62
    stop <- w121 stop-if-true
    # "Generate USER Event Loop"
    n30 = local read "Rising Edge"() -> (w117:bool)
    n31 = Or(x="OK Button", y=w117) -> (x .or. y?=w116:bool)
    n32 = local read "TASK ENABLE"() -> (w115:bool)
    n33 = And(x=w116, y=w115) -> (x .and. y?=w114:bool)
    n34 = case shown="True" w114 {
      selector: w114 -> [_ w141]
      tunnel: w130 -> [w140 w145]
      tunnel: [w140 w144] -> w127
      tunnel: w126 -> [w139 w143]
      tunnel: [w139 w142] -> w125
      frame False {
      }
      frame True {
        n35 = Generate User Event(user event=w145, event data cluster=w141, error in=w143) -> (user event out=w144:refnum<user-event>, error out=w142:errorcluster)  [unwired: 1 in]
      }
    }
    n36 = case shown="False" "STOP" {
      selector: "STOP" -> [_ w134]
      tunnel: w129 -> [w133 w138]
      tunnel: [w133 w137] -> w128
      tunnel: w124 -> [w132 w136]
      tunnel: [w132 w135] -> w123
      tunnel: [FALSE w134] -> w121
      frame False {
      }
      frame True {
        n37 = Generate User Event(user event=w138, event data cluster=w134, error in=w136) -> (user event out=w137:refnum<user-event>, error out=w135:errorcluster)  [unwired: 1 in]
      }
    }
    n38 = call "FGV Bool.vi"("Init/Read/Write State"=States_for_Action_Engine."Write", "Input Node"=w121) -> ()  [unwired: 1 in, 2 out]
    n39 = call "Wait4"("Count(uSec)"=u32 20) -> ()  [unwired: 1 out]
  }
  n40 = while {
    tunnel: w59 -> [w152]
    tunnel: [w151] -> w58
    tunnel: w46 -> [w149]
    tunnel: [w148] -> w57
    tunnel: w52 -> [w147]
    tunnel: [w146] -> w49
    stop <- w150 stop-if-true
    # "EVENT Handling Loop"
    n41 = event shown="[1] <Start Task>: User Event" {
      selector: w152 -> [_ _ _]
      dyn-events: [_ _ _] -> w151
      timeout: _ -> [_ _ _]
      tunnel: [FALSE FALSE w181] -> w150
      tunnel: w149 -> [w157 w166 w179]
      tunnel: [w156 w165 w180] -> w148
      tunnel: w147 -> [w155 w164 w178]
      tunnel: [w154 w163 w177] -> w146
      event Timeout {
        n42 = event-data() -> ()  [unwired: 1 in, 3 out]
        n43 = Enqueue Element(queue=w157, element=Intruction_Type_Definitions."None" ("Enum"), error in (no error)=w155) -> (queue out=w156:refnum<queue>, error out=w154:errorcluster)  [unwired: 1 in, 1 out]
      }
      event User Event {
        n44 = event-data() -> ()  [unwired: 1 in, 5 out]
        n45 = call "Arduino Interfacing VI.vi"("AE Mode"=Arduino_Interfacing."Read From Arduino") -> ("Arduino Data"=w160:T4)  [unwired: 3 in, 1 out]
        n46 = Unbundle By Name(w160) -> ("Rotary Switch"=w159:u8)
        n47 = case shown="9" w159 {
          tunnel: [Intruction_Type_Definitions."None" ("Enum") Intruction_Type_Definitions."Start Task 1" ("Enum") Intruction_Type_Definitions."Start Task 2" ("Enum") Intruction_Type_Definitions."Start Task 3" ("Enum") Intruction_Type_Definitions."Start Task 4" ("Enum") Intruction_Type_Definitions."Start Task 5" ("Enum") Intruction_Type_Definitions."Start Task 6" ("Enum") Intruction_Type_Definitions."Start Task 9" ("Enum")] -> w162
          frame 0, Default {
          }
          frame 1 {
          }
          frame 2 {
          }
          frame 3 {
          }
          frame 4 {
          }
          frame 5 {
          }
          frame 6 {
          }
          frame 9 {
          }
        }
        n48 = Enqueue Element(queue=w166, element=w162, error in (no error)=w164) -> (queue out=w165:refnum<queue>, error out=w163:errorcluster)  [unwired: 1 in, 1 out]
      }
      event User Event {
        n49 = event-data() -> ("Stop Queue"=w181:bool)  [unwired: 1 in, 4 out]
        n50 = Enqueue Element At Opposite End(queue=w179, element=Intruction_Type_Definitions."Exit" ("Enum"), error in (no error)=w178) -> (queue out=w180:refnum<queue>, error out=w177:errorcluster)  [unwired: 1 in, 1 out]
      }
    }
  }
  n51 = while {
    tunnel: w47 -> [w191]
    tunnel: w46 -> [w188]
    stop <- w185 stop-if-true
    # "Status Loop for Action Queues"
    n52 = Get Queue Status(queue=w191, return elements? (F)=TRUE) -> (error out=w187:errorcluster, # elements in queue=→"Action Queue Items":i32, elements=→"Action Queues items":string[])  [unwired: 1 in, 5 out]
    n53 = Get Queue Status(queue=w188, return elements? (F)=TRUE) -> (# pending remove=→"State Logic Queue Items":i32, error out=w186:errorcluster, elements=→"elements":T7[])  [unwired: 1 in, 5 out]
    n54 = Merge Errors(w187, w186) -> (w185:errorcluster)
    n55 = Wait (ms)(milliseconds to wait=u32 500) -> ()  [unwired: 1 out]
  }
  n56 = call "IMAQ Create"("Image Name"="Image dest") -> ("New Image"=w21:T23, "error out"=w20:errorcluster)  [unwired: 4 in]
  n57 = while {
    tunnel: w46 -> [w228]
    tunnel: w47 -> [w240]
    tunnel: w50 -> [w238]
    tunnel: [w237] -> _
    tunnel: [w236] -> w40
    shift-right: [w229] -> _
    shift-left: T15 {"PING_A"=0, "PING_B"=0, "PING_C"=0, "PING_D"=0} -> [w231]
    shift-right: [w222] -> _
    shift-left: State_Type_Definitions."Startup" ("Enum") -> [w225]
    shift-right: [w218] -> _
    shift-left: T16 {"xDistance"=0.0, "yDistance"=0.0, "wDistance"=0.0} -> [w220]
    shift-right: [w215] -> _
    shift-left: _ -> [w214]
    tunnel: w21 -> [w213]
    tunnel: w20 -> [w212]
    shift-right: [w209] -> _
    shift-left: T14 {"Recognized Object"=FALSE, "Object X coordinate"=0.0, "Object Y coordinate"=0.0} -> [w211]
    shift-right: [w206] -> _
    shift-left: T12 {"y Stepper Position"=0, "z Stepper Position"=0} -> [w208]
    shift-right: [w203] -> _
    shift-left: T11 {"Yaw"=0.0, "Compass"=0.0} -> [w205]
    shift-right: [w200] -> _
    shift-left: T10 {"Time up flag"=FALSE, "SET TIME TO CHECK"=0.0} -> [w202]
    shift-right: [w198] -> _
    shift-left: T9 {"yStepper desired"=0} -> [w199]
    shift-right: [w194] -> _
    shift-left: T8 {"Left IR Sensor"=0.0, "Arm IR Sensor"=0.0, "Bottom IR Sensor"=0.0} -> [w196]
    stop <- w227 stop-if-true
    # ">>> yStepper command>>>"
    # ">>True Stop Next State >>"
    # ">>Error  >>"
    # ">>Timeout>>"
    # ">>Action states Queue Reference >>"
    # ">>State Logic Queue Reference >>"
    # "TOP LEVEL BASELINE (MAIN PROCESSING LOOP)"
    n58 = Dequeue Element(queue=w240, timeout in ms (-1)=0, error in (no error)=w238) -> (queue out=w232:refnum<queue>, element=w239:string, error out=w233:errorcluster)  [unwired: 1 out]
    "Action State" <- w239
    n59 = Wait (ms)(milliseconds to wait=u32 20) -> ()  [unwired: 1 out]
    n60 = case shown="\"NAVX CALIBRATE\"" w239 {
      tunnel: [_ _ _ _ _ _ _ _ _ _ _ _ _ _ _ _ _ _ 0 w1600 _ _ _ _ _ _ _ _ _ _ _ _ _ _ _ _ _ _ _ _ _ _ _ _ _ _] -> w235
      tunnel: w232 -> [_ _ _ _ _ _ _ _ _ _ _ _ _ _ _ _ _ _ _ _ _ _ _ _ _ _ _ _ _ _ _ _ _ _ _ _ _ _ _ _ _ _ _ _ _ _]
      tunnel: w231 -> [w1371 w1380 w1392 w1403 w1420 w1431 w1442 w1454 w1466 w1477 w1484 w1499 w1513 w1525 w1533 w1545 w1570 w1580 w1591 w1601 w1610 w1620 w1650 w1661 w1669 w1678 w1691 w1704 w1714 w1723 w1740 w1749 w1760 w1770 w1780 w1790 w1797 w1809 w1825 w1831 w1843 w1855 w1867 w1879 w1891 w1902]
      tunnel: [w1371 w1380 w1392 w1403 w1420 w1431 w1442 w1454 w1466 w1477 w1484 w1499 w1514 w1525 w1533 w1545 w1571 w1580 w1591 w1601 w1610 w1620 w1649 w1661 w1669 w1678 w1691 w1704 w1714 w1723 w1740 w1749 w1760 w1770 w1780 w1790 w1797 w1809 w1825 w1831 w1843 w1855 w1867 w1879 w1891 w1902] -> w230
      tunnel: [TRUE TRUE _ _ _ _ _ _ _ _ _ _ _ _ _ _ _ _ _ _ _ _ _ _ _ _ _ _ _ _ _ _ _ _ _ _ _ _ _ _ _ _ _ _ _ _] -> w227
      tunnel: w225 -> [w1369 w1378 w1391 w1402 w1419 w1430 w1441 w1453 w1465 w1476 w1483 w1498 w1512 w1524 w1531 w1544 w1569 w1579 w1588 w1598 w1609 w1619 w1648 w1660 w1668 w1677 w1690 w1703 w1713 w1722 w1739 w1748 w1759 w1769 w1779 w1789 w1796 w1808 w1824 w1830 w1842 w1854 w1866 w1878 w1890 w1901]
      tunnel: [_ _ _ _ _ _ _ _ _ _ _ _ _ _ _ _ _ _ _ TRUE _ _ _ _ _ _ _ _ _ _ _ _ _ _ _ _ _ _ _ _ _ _ _ _ _ _] -> w224
      tunnel: [w1369 w1378 w1391 w1402 w1419 w1430 w1441 w1453 w1465 w1476 w1483 w1498 w1512 w1524 w1531 w1544 w1569 w1579 w1588 w1598 w1609 w1619 w1648 w1660 w1668 w1677 w1690 w1703 w1713 w1722 w1739 w1748 w1759 w1769 w1779 w1789 w1796 w1808 w1824 w1830 w1842 w1854 w1866 w1878 w1890 w1901] -> w223
      tunnel: w220 -> [w1368 w1377 w1390 w1405 w1418 w1429 w1440 w1452 w1464 w1475 w1485 w1497 w1511 w1526 w1535 w1546 w1568 w1581 w1587 w1597 w1611 w1621 w1638 w1659 w1671 w1679 w1692 w1705 w1715 w1724 w1741 w1751 w1762 w1772 w1782 w1792 w1799 w1811 w1827 w1833 w1845 w1857 w1869 w1881 w1893 w1904]
      tunnel: [w1368 w1377 w1390 w1405 w1418 w1429 w1440 w1452 w1464 w1475 w1485 w1496 w1511 w1526 w1535 w1546 w1567 w1581 w1587 w1597 w1611 w1621 w1637 w1659 w1671 w1679 w1692 w1705 w1715 w1724 w1741 w1751 w1762 w1772 w1782 w1792 w1799 w1811 w1827 w1833 w1845 w1857 w1869 w1881 w1893 w1904] -> w219
      tunnel: w213 -> [w1363 _ _ _ _ _ _ _ _ _ _ _ _ _ _ _ _ _ _ _ _ _ _ _ _ _ _ _ _ _ w1735 _ _ _ _ _ _ _ _ _ _ _ _ _ _ _]
      tunnel: w212 -> [_ _ _ _ _ _ _ _ _ _ _ _ _ _ _ _ _ _ _ _ _ _ _ _ _ _ _ _ w1707 _ w1737 w1747 _ _ _ _ _ _ _ _ _ _ _ _ _ _]
      tunnel: w211 -> [w1367 w1376 w1389 w1404 w1417 w1428 w1439 w1451 w1463 w1473 w1482 w1495 w1510 w1519 w1534 w1543 w1559 w1578 w1586 w1596 w1608 w1618 w1643 w1657 w1670 w1676 w1689 w1702 w1709 w1721 w1732 w1750 w1761 w1771 w1781 w1791 w1798 w1810 w1826 w1832 w1844 w1856 w1868 w1880 w1892 w1903]
      tunnel: [w1367 w1376 w1389 w1404 w1417 w1428 w1439 w1451 w1463 w1473 w1482 w1495 w1510 w1519 w1534 w1543 w1558 w1578 w1586 w1596 w1608 w1618 w1642 w1657 w1670 w1676 w1689 w1702 w1709 w1721 w1731 w1750 w1761 w1771 w1781 w1791 w1798 w1810 w1826 w1832 w1844 w1856 w1868 w1880 w1892 w1903] -> w210
      tunnel: w208 -> [w1366 w1375 w1388 w1406 w1416 w1427 w1438 w1450 w1462 w1472 w1481 w1494 w1509 w1527 w1536 w1542 w1564 w1577 w1585 w1595 w1607 w1617 w1633 w1656 w1667 w1675 w1688 w1701 w1712 w1720 w1742 w1752 w1758 w1768 w1778 w1788 w1800 w1812 w1823 w1834 w1846 w1858 w1870 w1882 w1894 w1905]
      tunnel: [w1366 w1375 w1388 w1406 w1416 w1427 w1438 w1450 w1462 w1472 w1481 w1494 w1509 w1527 w1536 w1542 w1563 w1577 w1585 w1595 w1607 w1617 w1632 w1656 w1667 w1675 w1688 w1701 w1712 w1720 w1742 w1752 w1758 w1768 w1778 w1788 w1800 w1812 w1822 w1834 w1846 w1858 w1870 w1882 w1894 w1905] -> w207
      tunnel: w205 -> [w1365 w1374 w1386 w1407 w1414 w1425 w1437 w1448 w1460 w1471 w1480 w1493 w1502 w1522 w1537 w1541 w1554 w1576 w1584 w1594 w1606 w1616 w1629 w1655 w1664 w1674 w1687 w1700 w1711 w1719 w1743 w1753 w1757 w1765 w1775 w1785 w1801 w1813 w1817 w1835 w1847 w1859 w1871 w1883 w1895 w1906]
      tunnel: [w1365 w1374 w1386 w1407 w1414 w1425 w1437 w1448 w1460 w1471 w1480 w1493 w1502 w1521 w1537 w1541 w1553 w1576 w1584 w1594 w1606 w1616 w1628 w1655 w1664 w1674 w1687 w1700 w1711 w1719 w1743 w1753 w1757 w1765 w1775 w1785 w1801 w1813 w1817 w1835 w1847 w1859 w1871 w1883 w1895 w1906] -> w204
      tunnel: w202 -> [w1362 w1373 w1387 w1408 w1415 w1426 w1436 w1449 w1461 w1470 w1479 w1492 w1501 w1518 w1538 w1540 w1550 w1573 w1583 w1593 w1605 w1615 w1626 w1653 w1663 w1673 w1686 w1699 w1710 w1718 w1744 w1754 w1756 w1764 w1774 w1784 w1802 w1814 w1816 w1829 w1841 w1853 w1865 w1877 w1889 w1900]
      tunnel: [w1362 w1373 w1387 w1408 w1415 w1426 w1436 w1449 w1461 w1470 w1479 w1492 w1501 w1518 w1538 w1540 w1550 w1573 w1583 w1593 w1605 w1615 w1625 w1653 w1663 w1673 w1686 w1699 w1710 w1718 w1744 w1754 w1756 w1764 w1774 w1784 w1802 w1814 w1816 w1829 w1839 w1851 w1863 w1875 w1887 w1899] -> w201
      tunnel: w199 -> [_ _ _ _ _ _ _ _ _ _ _ _ _ _ _ _ _ _ _ _ _ _ _ _ _ _ _ _ _ _ _ _ _ _ _ _ _ w1805 _ _ _ _ _ _ _ _]
      tunnel: [w1361 w1372 w1381 w1398 w1409 w1421 w1432 w1443 w1455 w1467 w1478 w1486 w1500 w1515 w1529 w1539 w1547 w1572 w1582 w1592 w1604 w1612 w1622 w1652 w1662 w1672 w1680 w1693 w1706 w1716 w1725 w1745 w1755 w1763 w1773 w1783 w1793 w1803 w1815 w1828 w1836 w1848 w1860 w1872 w1884 w1896] -> w195
      tunnel: w196 -> [w1361 w1372 w1381 w1398 w1409 w1421 w1432 w1443 w1455 w1467 w1478 w1486 w1500 w1515 w1530 w1539 w1547 w1572 w1582 w1592 w1604 w1612 w1622 w1652 w1662 w1672 w1680 w1693 w1706 w1716 w1725 w1745 w1755 w1763 w1773 w1783 w1793 w1803 w1815 w1828 w1836 w1848 w1860 w1872 w1884 w1896]
      frame "Exit" {
        # ">>State Logic  >>"
        # ">>> Time cluster >>>"
        # ">>> Yaw >>>"
        # ">>> Stepper position >>>"
        # ">>> Encoders >>>"
        # ">>> Object detection >>>"
        # ">>> Ultrasonic Sensors Detect >>>"
        n61 = call "Imaq Dispose"("All Images? (No)"=TRUE, "Image"=w1363) -> ()  [unwired: 4 in, 1 out]
      }
      frame "----Movement States----" {
        # ">>State Logic  >>"
        # ">>> Time cluster >>>"
        # ">>> Yaw >>>"
        # ">>> Stepper position >>>"
        # ">>> Encoders >>>"
        # ">>> Object detection >>>"
        # ">>> Ultrasonic Sensors Detect >>>"
      }
      frame "FORWARD" {
        # ">>State Logic  >>"
        # ">>> Time cluster >>>"
        # ">>> Yaw >>>"
        # ">>> Stepper position >>>"
        # ">>> Encoders >>>"
        # ">>> Object detection >>>"
        # ">>> Ultrasonic Sensors Detect >>>"
        n62 = Unbundle By Name(w1386) -> ("Yaw"=w1382:dbl)
        n63 = call "MOTOR CONTROL WITH PID AE.vi"("Yaw"=w1382, "Speed"=50.0, "Direction"=MOTOR_CONTROL_WITH_PID_AE_DIRECTION_TYPE_DEF."y-axis movement", "AE Mode"=MOTOR_CONTROL_WITH_PID_AE_DATA_MODE_TYPE_DEF."Write to AE") -> ()  [unwired: 1 out]
      }
      frame "FORWARD - IR ASSIST" {
        # ">>State Logic  >>"
        # ">>> Time cluster >>>"
        # ">>> Yaw >>>"
        # ">>> Stepper position >>>"
        # ">>> Encoders >>>"
        # ">>> Object detection >>>"
        # ">>> Ultrasonic Sensors Detect >>>"
        n64 = Unbundle By Name(w1398) -> ("Left IR Sensor"=w1397:dbl)
        n65 = Subtract(x=w1397, y=15.0) -> (x-y=w1395:dbl)
        n66 = Multiply(x=w1395, y=0.5) -> (x*y=w1393:dbl)
        n67 = call "MOTOR CONTROL WITH PID AE.vi"("Yaw"=w1393, "Speed"=30.0, "Direction"=MOTOR_CONTROL_WITH_PID_AE_DIRECTION_TYPE_DEF."y-axis movement", "AE Mode"=MOTOR_CONTROL_WITH_PID_AE_DATA_MODE_TYPE_DEF."Write to AE") -> ()  [unwired: 1 out]
      }
      frame "LEFT" {
        # ">>State Logic  >>"
        # ">>> Time cluster >>>"
        # ">>> Yaw >>>"
        # ">>> Stepper position >>>"
        # ">>> Encoders >>>"
        # ">>> Object detection >>>"
        # ">>> Ultrasonic Sensors Detect >>>"
        n68 = Unbundle By Name(w1414) -> ("Yaw"=w1411:dbl)
        n69 = call "MOTOR CONTROL WITH PID AE.vi"("Yaw"=w1411, "Speed"=-25.0, "Direction"=MOTOR_CONTROL_WITH_PID_AE_DIRECTION_TYPE_DEF."x-axis movement", "AE Mode"=MOTOR_CONTROL_WITH_PID_AE_DATA_MODE_TYPE_DEF."Write to AE") -> ()  [unwired: 1 out]
      }
      frame "R-ACW" {
        # ">>> IR Sensors >>>"
        # ">>> Time cluster >>>"
        # ">>> Yaw >>>"
        # ">>> Stepper position >>>"
        # ">>> Encoders >>>"
        # ">>> Object detection >>>"
        # ">>> Ultrasonic Sensors Detect >>>"
        n70 = call "MOTOR CONTROL WITH PID AE.vi"("Speed"=-10.0, "Direction"=MOTOR_CONTROL_WITH_PID_AE_DIRECTION_TYPE_DEF."rotation", "AE Mode"=MOTOR_CONTROL_WITH_PID_AE_DATA_MODE_TYPE_DEF."Write to AE") -> ()  [unwired: 1 in, 1 out]
      }
      frame "R-CW" {
        (unwired) -0.2 ("Speed")
        # ">>> Time cluster >>>"
        # ">>> Yaw >>>"
        # ">>> Stepper position >>>"
        # ">>> Encoders >>>"
        # ">>> Object detection >>>"
        # ">>> Ultrasonic Sensors Detect >>>"
        n71 = call "MOTOR CONTROL WITH PID AE.vi"("Speed"=10.0, "Direction"=MOTOR_CONTROL_WITH_PID_AE_DIRECTION_TYPE_DEF."rotation", "AE Mode"=MOTOR_CONTROL_WITH_PID_AE_DATA_MODE_TYPE_DEF."Write to AE") -> ()  [unwired: 1 in, 1 out]
      }
      frame "RIGHT" {
        # ">>> Time cluster >>>"
        # ">>> Yaw >>>"
        # ">>> Stepper position >>>"
        # ">>> Encoders >>>"
        # ">>> Object detection >>>"
        # ">>> Ultrasonic Sensors Detect >>>"
        n72 = Unbundle By Name(w1448) -> ("Yaw"=w1444:dbl)
        n73 = call "MOTOR CONTROL WITH PID AE.vi"("Yaw"=w1444, "Speed"=50.0, "Direction"=MOTOR_CONTROL_WITH_PID_AE_DIRECTION_TYPE_DEF."x-axis movement", "AE Mode"=MOTOR_CONTROL_WITH_PID_AE_DATA_MODE_TYPE_DEF."Write to AE") -> ()  [unwired: 1 out]
      }
      frame "REVERSE" {
        # ">>> Time cluster >>>"
        # ">>> Yaw >>>"
        # ">>> Stepper position >>>"
        # ">>> Encoders >>>"
        # ">>> Object detection >>>"
        # ">>> Ultrasonic Sensors Detect >>>"
        n74 = Unbundle By Name(w1460) -> ("Yaw"=w1456:dbl)
        n75 = call "MOTOR CONTROL WITH PID AE.vi"("Yaw"=w1456, "Speed"=-50.0, "Direction"=MOTOR_CONTROL_WITH_PID_AE_DIRECTION_TYPE_DEF."y-axis movement", "AE Mode"=MOTOR_CONTROL_WITH_PID_AE_DATA_MODE_TYPE_DEF."Write to AE") -> ()  [unwired: 1 out]
      }
      frame "STOP" {
        n76 = Wait (ms)(milliseconds to wait=u32 100) -> ()  [unwired: 1 out]
        n77 = call "MOTOR CONTROL WITH PID AE.vi"("Direction"=MOTOR_CONTROL_WITH_PID_AE_DIRECTION_TYPE_DEF."stop", "AE Mode"=MOTOR_CONTROL_WITH_PID_AE_DATA_MODE_TYPE_DEF."Write to AE") -> ()  [unwired: 2 in, 1 out]
      }
      frame "----SENSOR READING---- " {
      }
      frame "READ ENCODERS" {
        # ">>> Time cluster >>>"
        # ">>> Yaw >>>"
        # ">>> Stepper position >>>"
        # ">>> Object detection >>>"
        # ">>> Current encoder distance >>>"
        # ">>> Ultrasonic Sensors Detect >>>"
        n78 = call "MOTOR CONTROL WITH PID AE.vi"("AE Mode"=MOTOR_CONTROL_WITH_PID_AE_DATA_MODE_TYPE_DEF."Read from AE") -> ("Speed & distance"=w1490:T1)  [unwired: 3 in]
        n79 = Unbundle By Name(w1490) -> ("xDistance"=w1489:dbl, "yDistance"=w1488:dbl, "wDistance"=w1487:dbl)
        n80 = Bundle By Name(cluster=w1497, "xDistance"=w1489, "yDistance"=w1488, "wDistance"=w1487) -> (w1496:T16)
      }
      frame "READ ULTRASONIC" {
        (unwired) navX_type_def."Read Values" ("Mode")
        (unwired) MOTOR_CONTROL_NO_PID_Type_Def."Latch" ("Direction")
        # ">>State Logic  >>"
        # ">>> Time cluster >>>"
        # ">>> Ultrasonic Sensors Detect >>>"
        # ">>> Object detection >>>"
        # ">>> Encoders >>>"
        # ">>> Stepper position >>>"
        # ">>> Yaw >>>"
        n81 = call "Arduino Interfacing VI.vi"("AE Mode"=Arduino_Interfacing."Read From Arduino") -> ("Arduino Data"=w1507:T4)  [unwired: 3 in, 1 out]
        n82 = Unbundle By Name(w1507) -> ("PING A"=w1506:u8, "PING B"=w1505:u8, "PING C"=w1504:u8, "PING D"=w1503:u8)
        n83 = Bundle By Name(cluster=w1513, "PING_A"=w1506, "PING_B"=w1505, "PING_C"=w1504, "PING_D"=w1503) -> (w1514:T15)
      }
      frame "READ NAVX" {
        # ">>> Time cluster >>>"
        # ">>> Yaw >>>"
        # ">>> Ultrasonic Sensors Detect >>>"
        # ">>> Object detection >>>"
        # ">>> Encoders >>>"
        # ">>> Stepper position >>>"
        n84 = call "navX reading VI.vi"("Mode"=navX_type_def."Read Values") -> ("NavX Readings"=w1517:T3)  [unwired: 2 in, 3 out]
        n85 = Unbundle By Name(w1517) -> ("Heading"=w1516:dbl)
        n86 = Unbundle By Name(w1517) -> ("Yaw"=w1520:dbl)
        n87 = Bundle By Name(cluster=w1522, "Yaw"=w1520, "Compass"=w1516) -> (w1521:T11)
      }
      frame "READ IR" {
        w1532 = T33 [enum."A/AI0"] items=["Not Connected", "AudioIn/Left", "AudioIn/Right", "C/AI0", "C/AI1", "A/AI0", "A/AI1", "A/AI2", "A/AI3", "A/AI4", "A/AI5", "A/AI6", "A/AI7", "B/AI0", "B/AI1", "B/AI2", "B/AI3", "B/AI4", "B/AI5", "B/AI6", "B/AI7", "AI/AI0", "AI/AI1", "AI/AI2", "AI/AI3", "A/AI0 (DIFF)", "A/AI1 (DIFF)", "A/AI2 (DIFF)", "A/AI3 (DIFF)", "B/AI0 (DIFF)", "B/AI1 (DIFF)", "B/AI2 (DIFF)", "B/AI3 (DIFF)"] ("AI Channel")
        # ">>State Logic  >>"
        # ">>> Time cluster >>>"
        # ">>> Ultrasonic Sensors Detect >>>"
        # ">>> Object detection >>>"
        # ">>> Encoders >>>"
        # ">>> Stepper position >>>"
        # ">>> Yaw >>>"
        n88 = call <vilib>:"Sharp IR.vi"("AI Channel"=w1532) -> ("Sharp IR Distance"=w1528:dbl)  [unwired: 8 in, 2 out]
        n89 = Bundle By Name(cluster=w1530, "Left IR Sensor"=w1528) -> (w1529:T8)
      }
      frame "----SYSTEM MODES----" {
        (unwired) I2C_MASTER_Type_Def."Last State" ("Arduino Mode")
        # ">>> Object detection >>>"
        # ">>> Yaw >>>"
        # ">>> Ultrasonic Sensors Detect >>>"
        # ">>> Encoders >>>"
        # ">>> Stepper position >>>"
      }
      frame "INIT" {
        w1565 = u8 0
        w1566 = 0.0
        # ">>> Time cluster >>>"
        # ">>> Object detection >>>"
        # ">>> Yaw >>>"
        # ">>> Ultrasonic Sensors Detect >>>"
        # ">>> Encoders >>>"
        # ">>> Stepper position >>>"
        # ">>State Logic  >>"
        n90 = call "Arduino Interfacing VI.vi"("AE Mode"=Arduino_Interfacing."Initialize") -> ()  [unwired: 3 in, 2 out]
        n91 = call "FGV Bool.vi"("Init/Read/Write State"=States_for_Action_Engine."Initialize") -> ()  [unwired: 2 in, 2 out]
        n92 = call "Elasped Timer.vi"("Action"=Elapsed_timer_control."Initialize") -> ()  [unwired: 7 in, 4 out]
        n93 = call "MOTOR CONTROL WITH PID AE.vi"("AE Mode"=MOTOR_CONTROL_WITH_PID_AE_DATA_MODE_TYPE_DEF."Init AE") -> ()  [unwired: 3 in, 1 out]
        n94 = Bundle By Name(cluster=w1559, "Recognized Object"=FALSE, "Object X coordinate"=0.0, "Object Y coordinate"=0.0) -> (w1558:T14)
        n95 = Bundle By Name(cluster=w1564, "y Stepper Position"=u8 0, "z Stepper Position"=u8 0) -> (w1563:T12)
        n96 = Bundle By Name(cluster=w1568, "xDistance"=w1566, "yDistance"=w1566, "wDistance"=w1566) -> (w1567:T16)
        n97 = Bundle By Name(cluster=w1570, "PING_A"=w1565, "PING_B"=w1565, "PING_C"=w1565, "PING_D"=w1565) -> (w1571:T15)
        n98 = Bundle By Name(cluster=w1554, "Yaw"=0.0) -> (w1553:T11)
      }
      frame "ARDUINO - ULTRASONIC" {
        # ">>> Object detection >>>"
        # ">>> Yaw >>>"
        # ">>> Ultrasonic Sensors Detect >>>"
        # ">>> Encoders >>>"
        # ">>> Stepper position >>>"
        # ">>State Logic  >>"
        n99 = call "Arduino Interfacing VI.vi"("Data to Write"=I2C_MASTER_WRITE_NEW_Type_Def."Ultrasonic sensors", "AE Mode"=Arduino_Interfacing."Write to Arduino") -> ()  [unwired: 2 in, 2 out]
      }
      frame "NAVX CALIBRATE" {
        # ">>> Object detection >>>"
        # ">>> Yaw >>>"
        # ">>> Ultrasonic Sensors Detect >>>"
        # ">>> Encoders >>>"
        # ">>> Stepper position >>>"
        # ">>State Logic  >>"
        # "Adds a 15 second delay to the startup process \nfor the NavX to calibrate"
        n100 = Wait (ms)(milliseconds to wait=u32 1000) -> ()  [unwired: 1 out]
      }
      frame "NO ACTION", Default {
        (unwired) u8 0 ("y Stepper value")
        (unwired) TRUE ("Latch")
        (unwired) navX_type_def."Read Values" ("Mode")
        (unwired) MOTOR_CONTROL_NO_PID_Type_Def."Latch" ("Direction")
        # ">>> Object detection >>>"
        # ">>> Yaw >>>"
        # ">>> Ultrasonic Sensors Detect >>>"
        # ">>> Encoders >>>"
        # ">>> Stepper position >>>"
        # ">>State Logic  >>"
        n101 = case shown="4" w1598 {
          tunnel: [0 100] -> w1600
          frame 1, Default {
          }
          frame 4 {
          }
        }
      }
      frame "----RESET CASES----" {
        (unwired) I2C_MASTER_Type_Def."Last State" ("Arduino Mode")
        # ">>> Object detection >>>"
        # ">>> Yaw >>>"
        # ">>> Ultrasonic Sensors Detect >>>"
        # ">>> Encoders >>>"
        # ">>> Stepper position >>>"
        # ">>State Logic  >>"
      }
      frame "RESET ENCODERS" {
        # ">>> Object detection >>>"
        # ">>> Yaw >>>"
        # ">>> Ultrasonic Sensors Detect >>>"
        # ">>> Encoders >>>"
        # ">>> Stepper position >>>"
        # ">>State Logic  >>"
        n102 = call "MOTOR CONTROL WITH PID AE.vi"("Direction"=MOTOR_CONTROL_WITH_PID_AE_DIRECTION_TYPE_DEF."reset encoders", "AE Mode"=MOTOR_CONTROL_WITH_PID_AE_DATA_MODE_TYPE_DEF."Write to AE") -> ()  [unwired: 2 in, 1 out]
      }
      frame "RESET FLAGS" {
        (unwired) I2C_MASTER_Type_Def."Last State" ("Arduino Mode")
        # "Resets any software variables\nand/or non-critical states"
        n103 = Wait (ms)(milliseconds to wait=u32 20) -> ()  [unwired: 1 out]
        n104 = Bundle By Name(cluster=w1626, "Time up flag"=FALSE, "SET TIME TO CHECK"=0.0) -> (w1625:T10)
        n105 = Bundle By Name(cluster=w1643, "Recognized Object"=FALSE, "Object X coordinate"=0.0, "Object Y coordinate"=0.0) -> (w1642:T14)
        n106 = Bundle By Name(cluster=w1633, "y Stepper Position"=u8 0, "z Stepper Position"=u8 0) -> (w1632:T12)
        n107 = Bundle By Name(cluster=w1638, "xDistance"=0.0, "yDistance"=0.0, "wDistance"=0.0) -> (w1637:T16)
        n108 = Bundle By Name(cluster=w1650, "PING_A"=u8 0, "PING_B"=u8 0, "PING_C"=u8 0, "PING_D"=u8 0) -> (w1649:T15)
        n109 = Bundle By Name(cluster=w1629, "Yaw"=0.0) -> (w1628:T11)
      }
      frame "RESET YAW" {
        n110 = Wait (ms)(milliseconds to wait=u32 100) -> ()  [unwired: 1 out]
        n111 = call "navX reading VI.vi"("Mode"=navX_type_def."Zero Yaw") -> ()  [unwired: 2 in, 4 out]
      }
      frame "RESET ARM" {
        n112 = call "Arduino Interfacing VI.vi"("Data to Write"=I2C_MASTER_WRITE_NEW_Type_Def."Soft Reset", "AE Mode"=Arduino_Interfacing."Write to Arduino") -> ()  [unwired: 2 in, 2 out]
      }
      frame "--------CAM STATES-------" {
      }
      frame "OPEN LOG CAM" {
        n113 = call "Webcam AE.vi"("Session In"=T30 "cam0", "Camera states"=Webcam_AE."Initialize Camera") -> ("error out"=w1683:errorcluster, "Session Out"=w1682:T30)  [unwired: 1 in, 1 out]
        n114 = call "Webcam AE.vi"("error in (no error)"=w1683, "Session In"=w1682, "Camera states"=Webcam_AE."Open Camera") -> ()  [unwired: 3 out]
      }
      frame "OPEN LIFE CAM" {
        n115 = call "Webcam AE.vi"("Session In"=T30 "cam1", "Camera states"=Webcam_AE."Initialize Camera") -> ("error out"=w1696:errorcluster, "Session Out"=w1695:T30)  [unwired: 1 in, 1 out]
        n116 = call "Webcam AE.vi"("error in (no error)"=w1696, "Session In"=w1695, "Camera states"=Webcam_AE."Open Camera") -> ()  [unwired: 3 out]
      }
      frame "CAM ACQ" {
        # ">>State Logic  >>"
        # ">>> Time cluster >>>"
        # ">>> Yaw >>>"
        # ">>> Stepper position >>>"
        # ">>> Encoders >>>"
        # ">>> Object detection >>>"
        # ">>> Ultrasonic Sensors Detect >>>"
        n117 = call "Webcam AE.vi"("error in (no error)"=w1707, "Camera states"=Webcam_AE."Continuous Acquisition") -> ()  [unwired: 1 in, 3 out]
      }
      frame "CAM CLOSE" {
        # ">>State Logic  >>"
        # ">>> Time cluster >>>"
        # ">>> Yaw >>>"
        # ">>> Stepper position >>>"
        # ">>> Encoders >>>"
        # ">>> Object detection >>>"
        # ">>> Ultrasonic Sensors Detect >>>"
        n118 = call "Webcam AE.vi"("Camera states"=Webcam_AE."Close Camera") -> ()  [unwired: 2 in, 3 out]
      }
      frame "PROCESS IMAGE" {
        # ">>State Logic  >>"
        # ">>> Time cluster >>>"
        # ">>> Yaw >>>"
        # ">>> Stepper position >>>"
        # ">>> Encoders >>>"
        # ">>> Object detection >>>"
        # ">>> Ultrasonic Sensors Detect >>>"
        n119 = call "Webcam AE.vi"("error in (no error)"=w1737, "Camera states"=Webcam_AE."Retrieve Image") -> ("error out"=w1733:errorcluster, "Image Out"=w1736:T23)  [unwired: 1 in, 1 out]
        n120 = call "Object Detection SubVI.vi"("Error In"=w1733, "Mode"="Object recognition mode", "Image Dest"=w1735, "Image in"=w1736) -> ("Object Center Coordinates"=w1730:cluster{"x":sgl, "y":sgl}, "Object detection cluster"=w1726:T2)  [unwired: 2 out]
        "Object detection cluster" <- w1726
        "Object Center Coordinates" <- w1730
        n121 = Unbundle By Name(w1726) -> ("Object detected?"=w1727:bool)
        n122 = Unbundle By Name(w1730) -> ("x"=w1729:sgl, "y"=w1728:sgl)
        n123 = Bundle By Name(cluster=w1732, "Recognized Object"=w1727, "Object X coordinate"=w1729, "Object Y coordinate"=w1728) -> (w1731:T14)
      }
      frame "DISPOSE BUFFERS" {
        # ">>State Logic  >>"
        # ">>> Time cluster >>>"
        # ">>> Yaw >>>"
        # ">>> Stepper position >>>"
        # ">>> Encoders >>>"
        # ">>> Object detection >>>"
        # ">>> Ultrasonic Sensors Detect >>>"
        n124 = call "Webcam AE.vi"("error in (no error)"=w1747, "Camera states"=Webcam_AE."Dispose Image Buffers") -> ()  [unwired: 1 in, 3 out]
      }
      frame "-----ARM ACTIONS-----" {
      }
      frame "CLOSE CLAW" {
        n125 = call "Arduino Interfacing VI.vi"("Data to Write"=I2C_MASTER_WRITE_NEW_Type_Def."Close Claw", "AE Mode"=Arduino_Interfacing."Write to Arduino") -> ()  [unwired: 2 in, 2 out]
      }
      frame "OPEN CLAW" {
        n126 = call "Arduino Interfacing VI.vi"("Data to Write"=I2C_MASTER_WRITE_NEW_Type_Def."Open Claw", "AE Mode"=Arduino_Interfacing."Write to Arduino") -> ()  [unwired: 2 in, 2 out]
      }
      frame "Z STEPPER CAM HEIGHT" {
        n127 = call "Arduino Interfacing VI.vi"("Data to Write"=I2C_MASTER_WRITE_NEW_Type_Def."zStepper 6k", "AE Mode"=Arduino_Interfacing."Write to Arduino") -> ()  [unwired: 2 in, 2 out]
      }
      frame "Z STEPPER GRAB HEIGHT" {
        # ">>State Logic  >>"
        # ">>> Time cluster >>>"
        # ">>> Yaw >>>"
        # ">>> Stepper position >>>"
        # ">>> Encoders >>>"
        # ">>> Object detection >>>"
        # ">>> Ultrasonic Sensors Detect >>>"
        n128 = call "Arduino Interfacing VI.vi"("Data to Write"=I2C_MASTER_WRITE_NEW_Type_Def."zStepper 100", "AE Mode"=Arduino_Interfacing."Write to Arduino") -> ()  [unwired: 2 in, 2 out]
      }
      frame "Y STEPPER CONTROL" {
        # ">>State Logic  >>"
        # ">>> yStepper command>>>"
        # ">>> Time cluster >>>"
        # ">>> Yaw >>>"
        # ">>> Stepper position >>>"
        # ">>> Encoders >>>"
        # ">>> Object detection >>>"
        # ">>> Ultrasonic Sensors Detect >>>"
        n129 = Unbundle By Name(w1805) -> ("yStepper desired"=w1804:u8)
        n130 = call "Arduino Interfacing VI.vi"("y Stepper value"=w1804, "Data to Write"=I2C_MASTER_WRITE_NEW_Type_Def."yStepper control", "AE Mode"=Arduino_Interfacing."Write to Arduino") -> ()  [unwired: 1 in, 2 out]
      }
      frame "READ STEPPER VALUES" {
        # ">>State Logic  >>"
        # ">>> Time cluster >>>"
        # ">>> Yaw >>>"
        # ">>> Stepper position >>>"
        # ">>> Encoders >>>"
        # ">>> Object detection >>>"
        # ">>> Ultrasonic Sensors Detect >>>"
        n131 = call "Arduino Interfacing VI.vi"("AE Mode"=Arduino_Interfacing."Read From Arduino") -> ("Arduino Data"=w1820:T4)  [unwired: 3 in, 1 out]
        n132 = Unbundle By Name(w1820) -> ("y Stepper Position"=w1819:u8, "z Stepper Position"=w1818:u8)
        n133 = Bundle By Name(cluster=w1823, "y Stepper Position"=w1819, "z Stepper Position"=w1818) -> (w1822:T12)
      }
      frame " -----TIMING-----" {
        # ">>State Logic  >>"
        # ">>> Time cluster >>>"
        # ">>> Yaw >>>"
        # ">>> Stepper position >>>"
        # ">>> Encoders >>>"
        # ">>> Object detection >>>"
        # ">>> Ultrasonic Sensors Detect >>>"
      }
      frame "SET TIMER 1" {
        # ">>State Logic  >>"
        # ">>> Time cluster >>>"
        # ">>> Yaw >>>"
        # ">>> Stepper position >>>"
        # ">>> Encoders >>>"
        # ">>> Object detection >>>"
        # ">>> Ultrasonic Sensors Detect >>>"
        n134 = call "Elasped Timer.vi"("Time Setting"=1.0, "Action"=Elapsed_timer_control."Initialize") -> ()  [unwired: 6 in, 4 out]
        n135 = Bundle By Name(cluster=w1841, "Time up flag"=FALSE) -> (w1839:T10)
      }
      frame "SET TIMER 2" {
        # ">>State Logic  >>"
        # ">>> Time cluster >>>"
        # ">>> Yaw >>>"
        # ">>> Stepper position >>>"
        # ">>> Encoders >>>"
        # ">>> Object detection >>>"
        # ">>> Ultrasonic Sensors Detect >>>"
        n136 = call "Elasped Timer.vi"("Time Setting"=2.0, "Action"=Elapsed_timer_control."Initialize") -> ()  [unwired: 6 in, 4 out]
        n137 = Bundle By Name(cluster=w1853, "Time up flag"=FALSE) -> (w1851:T10)
      }
      frame "SET TIMER 3" {
        # ">>State Logic  >>"
        # ">>> Time cluster >>>"
        # ">>> Yaw >>>"
        # ">>> Stepper position >>>"
        # ">>> Encoders >>>"
        # ">>> Object detection >>>"
        # ">>> Ultrasonic Sensors Detect >>>"
        n138 = call "Elasped Timer.vi"("Time Setting"=3.0, "Action"=Elapsed_timer_control."Initialize") -> ()  [unwired: 6 in, 4 out]
        n139 = Bundle By Name(cluster=w1865, "Time up flag"=FALSE) -> (w1863:T10)
      }
      frame "SET TIMER 4" {
        # ">>State Logic  >>"
        # ">>> Time cluster >>>"
        # ">>> Yaw >>>"
        # ">>> Stepper position >>>"
        # ">>> Encoders >>>"
        # ">>> Object detection >>>"
        # ">>> Ultrasonic Sensors Detect >>>"
        n140 = call "Elasped Timer.vi"("Time Setting"=4.0, "Action"=Elapsed_timer_control."Initialize") -> ()  [unwired: 6 in, 4 out]
        n141 = Bundle By Name(cluster=w1877, "Time up flag"=FALSE) -> (w1875:T10)
      }
      frame "SET TIMER 5" {
        # ">>State Logic  >>"
        # ">>> Time cluster >>>"
        # ">>> Yaw >>>"
        # ">>> Stepper position >>>"
        # ">>> Encoders >>>"
        # ">>> Object detection >>>"
        # ">>> Ultrasonic Sensors Detect >>>"
        n142 = call "Elasped Timer.vi"("Time Setting"=5.0, "Action"=Elapsed_timer_control."Initialize") -> ()  [unwired: 6 in, 4 out]
        n143 = Bundle By Name(cluster=w1889, "Time up flag"=FALSE) -> (w1887:T10)
      }
      frame "START TIMER" {
        # ">>State Logic  >>"
        # ">>> Time cluster >>>"
        # ">>> Yaw >>>"
        # ">>> Stepper position >>>"
        # ">>> Encoders >>>"
        # ">>> Object detection >>>"
        # ">>> Ultrasonic Sensors Detect >>>"
        n144 = call "Elasped Timer.vi"("Action"=Elapsed_timer_control."Start") -> ("Time Out?!"=w1897:bool)  [unwired: 7 in, 3 out]
        n145 = Bundle By Name(cluster=w1900, "Time up flag"=w1897) -> (w1899:T10)
      }
    }
    "State Logic" <- w223
    n146 = local read "TASK ENABLE"() -> (w217:bool)
    n147 = Not(x=w217) -> (.not. x?=w216:bool)
    n148 = case shown="True" w224 {
      tunnel: w228 -> [w252 w285]
      tunnel: w232 -> [w248 w287]
      tunnel: [w252 w285] -> w237
      tunnel: [w248 w288] -> w236
      tunnel: w233 -> [_ w283]
      tunnel: w235 -> [_ w284]
      tunnel: w230 -> [w251 w290]
      tunnel: [w251 w290] -> w229
      tunnel: "STOP TASK" -> [_ w273]
      tunnel: w223 -> [w250 w289]
      tunnel: [w250 w286] -> w222
      tunnel: w219 -> [w249 w279]
      tunnel: [w249 w279] -> w218
      tunnel: w216 -> [_ w274]
      tunnel: [w247 w271] -> w215
      tunnel: w214 -> [w247 w270]
      tunnel: w210 -> [w246 w267]
      tunnel: [w246 w267] -> w209
      tunnel: w207 -> [w245 w263]
      tunnel: [w245 w263] -> w206
      tunnel: w204 -> [w244 w261]
      tunnel: [w244 w261] -> w203
      tunnel: w201 -> [w243 w259]
      tunnel: [w243 w259] -> w200
      tunnel: w199 -> [w242 w258]
      tunnel: [w242 w257] -> w198
      tunnel: [_ w255] -> w197
      tunnel: w195 -> [w241 w253]
      tunnel: [w241 w253] -> w194
      frame False {
        # ">>> IR Sensors >>>"
        # ">>> IR Sensors >>>"
        # ">>> yStepper command>>>"
        # ">>> Time cluster >>>"
        # ">>> Yaw >>>"
        # ">>> Stepper position >>>"
        # ">>> Encoders >>>"
        # ">>> Object detection >>>"
        # ">>> Ultrasonic Sensors Detect >>>"
        # ">>> Time cluster >>>"
        # ">>> Yaw >>>"
        # ">>> Stepper position >>>"
        # ">>> Encoders >>>"
        # ">>> Object detection >>>"
        # ">>> Ultrasonic Sensors Detect >>>"
      }
      frame True {
        # ">>State Logic Queue Reference >>"
        # ">>Timeout>>"
        # ">>> yStepper command>>>"
        # ">>> Time cluster >>>"
        # ">>> Object detection >>>"
        # ">>> Yaw >>>"
        # ">>> Ultrasonic Sensors Detect >>>"
        # ">>> Encoders >>>"
        # ">>> Stepper position >>>"
        # ">>State Logic  >>"
        # ">>True Stop Next State >>"
        # ">>Action Queue>>"
        # ">> Manual override >>"
        # ">>> Time cluster >>>"
        # ">>> Yaw >>>"
        # ">>> Stepper position >>>"
        # ">>> Encoders >>>"
        # ">>> Object detection >>>"
        # ">>> Ultrasonic Sensors Detect >>>"
        # ">>Action Queue>>"
        # ">>State Logic Queue Reference >>"
        n149 = Or(x=w273, y=w274) -> (x .or. y?=w272:bool)
        n150 = Unbundle By Name(w253) -> ("Left IR Sensor"=w254:dbl)
        "Left IR Sensor" <- w254
        n151 = Unbundle By Name(w259) -> ("Time up flag"=w260:bool)
        "Time up flag" <- w260
        n152 = Unbundle By Name(w261) -> ("Yaw"=w262:dbl, "Compass"=w256:dbl)
        n153 = Unbundle By Name(w263) -> ("y Stepper Position"=w265:u8, "z Stepper Position"=w264:u8)
        n154 = Unbundle By Name(w279) -> ("xDistance"=w276:dbl, "yDistance"=w277:dbl, "wDistance"=w278:dbl)
        n155 = Unbundle By Name(w267) -> ("Recognized Object"=w266:bool, "Object X coordinate"=w269:dbl, "Object Y coordinate"=w268:dbl)
        n156 = Unbundle By Name(w290) -> ("PING_A"=w282:u8, "PING_B"=w281:u8, "PING_C"=w280:u8, "PING_D"=w275:u8)
        n157 = case shown="23" w289 {
          tunnel: [w293 w299 w311 w320 w387 w400 w435 w487 w528 w574 w616 w669 w715 w754 w813 w857 w901 w940 w987 w1028 w1079 w1115 w1163 w1205 w1235 w1282 w1322] -> w288
          tunnel: w287 -> [w293 w302 w312 w323 w389 w401 w444 w485 w532 w575 w622 w662 w718 w761 w803 w847 w904 w946 w986 w1031 w1069 w1121 w1158 w1196 w1239 w1289 w1327]
          tunnel: [State_Type_Definitions."Idle" ("Enum") State_Type_Definitions."Idle" ("Enum") w307 w322 State_Type_Definitions."Shutdown" ("Enum") w402 w442 w488 w529 w573 w617 w668 w716 w756 w812 w856 w902 w947 w988 w1030 w1078 w1122 w1164 w1197 w1236 w1283 w1323] -> w286
          tunnel: w285 -> [_ _ w310 w326 _ w407 w438 w484 w533 w582 w621 w666 w719 w760 w810 w854 w899 w945 w984 w1032 w1076 w1120 w1161 w1204 w1243 w1288 w1330]
          tunnel: w284 -> [_ _ _ w325 _ w406 w437 w483 w534 w581 w620 w665 w712 w759 w809 w853 w898 w944 w983 w1033 w1075 w1119 w1160 w1202 w1238 w1287 w1329]
          tunnel: w283 -> [_ _ w309 w321 _ w405 w436 w482 w535 w580 w619 w664 w711 w758 w811 w855 w900 w943 w982 w1034 w1077 w1118 w1159 w1203 w1242 w1286 w1328]
          tunnel: w272 -> [_ _ _ _ _ w399 w443 w481 w536 w577 w615 w667 w717 w762 w804 w848 w905 w941 w985 w1035 w1070 w1116 w1162 w1200 w1241 w1281 w1326]
          tunnel: w282 -> [_ _ _ _ _ _ _ _ _ _ _ _ _ _ _ _ _ _ _ _ _ _ _ _ _ _ _]
          tunnel: w281 -> [_ _ _ _ _ _ _ w480 _ _ _ w658 w700 w752 _ _ w891 _ _ _ _ _ _ _ _ _ _]
          tunnel: w280 -> [_ _ _ _ _ _ _ w479 _ _ _ w659 w701 w753 _ _ w892 _ _ _ _ _ _ _ _ _ _]
          tunnel: w278 -> [_ _ _ _ _ _ _ _ _ w579 _ _ _ _ _ _ _ _ _ _ _ _ _ _ _ _ _]
          tunnel: w277 -> [_ _ _ _ _ w398 _ _ w527 _ _ _ _ w757 _ _ _ _ _ _ _ _ _ _ _ _ _]
          tunnel: w276 -> [_ _ _ _ _ _ _ _ _ _ _ _ w706 _ _ _ _ _ _ _ _ _ _ _ _ _ _]
          tunnel: w275 -> [_ _ _ _ _ _ _ _ _ _ _ _ _ _ _ _ _ _ _ _ _ _ _ _ _ _ _]
          tunnel: [State_Type_Definitions."Idle" ("Enum") State_Type_Definitions."Idle" ("Enum") State_Type_Definitions."Idle" ("Enum") State_Type_Definitions."Idle" ("Enum") State_Type_Definitions."Shutdown" ("Enum") w395 w441 w486 w530 w570 w614 w661 w714 w755 w814 w858 w903 w939 w989 w1029 w1080 w1114 w1165 w1198 w1237 w1284 w1325] -> w271
          tunnel: w270 -> [_ _ w307 _ _ _ _ _ _ _ _ _ _ _ _ _ _ _ _ _ _ _ _ _ _ _ _]
          tunnel: w266 -> [_ _ _ _ _ _ _ _ _ _ _ _ _ _ _ _ _ _ _ _ _ _ _ w1199 _ _ _]
          tunnel: w269 -> [_ _ _ _ _ _ _ _ _ _ _ _ _ _ _ _ _ _ _ _ _ _ _ _ _ _ _]
          tunnel: w268 -> [_ _ _ _ _ _ _ _ _ _ _ _ _ _ _ _ _ _ _ w1024 _ _ _ _ _ _ _]
          tunnel: w265 -> [_ _ _ _ _ _ _ _ _ _ _ _ _ _ _ _ _ _ _ w1023 _ _ _ _ _ _ _]
          tunnel: w264 -> [_ _ _ _ _ _ w440 _ _ _ w612 _ _ _ w807 w851 _ _ _ _ w1073 _ w1157 _ w1240 _ _]
          tunnel: w262 -> [_ _ _ _ _ _ _ _ _ _ _ _ _ _ _ _ _ _ _ _ _ _ _ _ _ _ _]
          tunnel: w260 -> [_ _ _ _ _ _ _ _ _ _ _ _ _ _ _ _ _ w937 w979 _ _ w1112 _ _ _ _ _]
          tunnel: w258 -> [w291 w297 w306 w318 w385 w394 w439 w478 w531 w569 w613 w660 w710 w751 w802 w846 w896 w938 w980 w1026 w1068 w1113 w1154 w1195 w1234 w1285 w1324]
          tunnel: [w291 w296 w306 w318 w385 w394 w439 w478 w531 w569 w613 w660 w710 w751 w802 w846 w896 w938 w980 w1025 w1068 w1113 w1154 w1195 w1234 w1285 w1324] -> w257
          tunnel: w256 -> [_ _ _ _ _ _ _ _ _ _ _ _ _ _ _ _ _ _ _ _ _ _ _ _ _ w1280 _]
          tunnel: [_ _ _ TRUE _ _ _ _ _ _ _ _ _ _ _ _ _ _ _ _ _ _ _ _ _ _ _] -> w255
          tunnel: w254 -> [_ _ _ _ _ _ _ _ _ _ _ _ _ _ _ _ _ _ _ _ _ _ _ _ _ _ _]
          frame 0 {
            # ">>> yStepper command>>>"
          }
          frame 1 {
            # ">>> yStepper command>>>"
            n158 = for {
              shift-right: [w305] -> w299
              shift-left: w302 -> [w304]
              tunnel: string[] ["INIT", "RESET ARM", "RESET FLAGS", "RESET YAW", "NAVX CALIBRATE"] -> [w303] mode=indexing
              n159 = Enqueue Element(queue=w304, element=w303) -> (queue out=w305:refnum<queue>)  [unwired: 2 in, 2 out]
            }
            n160 = Bundle By Name(cluster=w297, "yStepper desired"=u8 0) -> (w296:T9)
          }
          frame 3 {
            # ">>> yStepper command>>>"
            n161 = Flush Queue(queue=w310, error in (no error)=w309) -> ()  [unwired: 3 out]
            n162 = for {
              shift-right: [w316] -> w311
              shift-left: w312 -> [w315]
              tunnel: string[] ["STOP", "RESET ENCODERS", "RESET YAW", "RESET ARM", "RESET FLAGS", "DISPOSE BUFFERS", "CAM CLOSE"] -> [w314] mode=indexing
              n163 = Enqueue Element(queue=w315, element=w314) -> (queue out=w316:refnum<queue>)  [unwired: 2 in, 2 out]
            }
          }
          frame 4, Default {
            (unwired) TRUE ("Green LED")
            # ">>> yStepper command>>>"
            n164 = Dequeue Element(queue=w326, timeout in ms (-1)=w325, error in (no error)=w321) -> (element=w324:T7)  [unwired: 3 out]
            n165 = case shown="\"Start Task 5\"" w324 {
              tunnel: [w328 w335 w342 w349 w356 w363 w370 w372 w380] -> w320
              tunnel: w323 -> [w329 w336 w343 w350 w357 w364 w370 w373 w379]
              tunnel: [State_Type_Definitions."Task 1" ("Enum") State_Type_Definitions."Task 2:Raise Arm" ("Enum") State_Type_Definitions."Task 3" ("Enum") State_Type_Definitions."Task 4_A" ("Enum") State_Type_Definitions."Task 5A: ARM CAM HEIGHT" ("Enum") State_Type_Definitions."Task 6_A" ("Enum") State_Type_Definitions."Idle" ("Enum") State_Type_Definitions."Shutdown" ("Enum") State_Type_Definitions."Task 9A: Raise Arm" ("Enum")] -> w322
              frame "Start Task 1" {
                n166 = for {
                  shift-right: [w333] -> w328
                  shift-left: w329 -> [w332]
                  tunnel: string[] ["RESET ENCODERS", "RESET YAW", "FORWARD", "READ ENCODERS"] -> [w331] mode=indexing
                  n167 = Enqueue Element(queue=w332, element=w331) -> (queue out=w333:refnum<queue>)  [unwired: 2 in, 2 out]
                }
              }
              frame "Start Task 2" {
                n168 = for {
                  shift-right: [w340] -> w335
                  shift-left: w336 -> [w339]
                  tunnel: string[] ["RESET ENCODERS", "RESET YAW", "READ ULTRASONIC", "ARDUINO - ULTRASONIC"] -> [w338] mode=indexing
                  n169 = Enqueue Element(queue=w339, element=w338) -> (queue out=w340:refnum<queue>)  [unwired: 2 in, 2 out]
                }
              }
              frame "Start Task 3" {
                n170 = for {
                  shift-right: [w347] -> w342
                  shift-left: w343 -> [w346]
                  tunnel: string[] ["RESET ENCODERS", "READ ENCODERS", "R-ACW"] -> [w345] mode=indexing
                  n171 = Enqueue Element(queue=w346, element=w345) -> (queue out=w347:refnum<queue>)  [unwired: 2 in, 2 out]
                }
              }
              frame "Start Task 4" {
                n172 = for {
                  shift-right: [w354] -> w349
                  shift-left: w350 -> [w353]
                  tunnel: string[] ["RESET YAW", "RESET ENCODERS", "RESET ARM", "RESET FLAGS", "", ""] -> [w352] mode=indexing
                  n173 = Enqueue Element(queue=w353, element=w352) -> (queue out=w354:refnum<queue>)  [unwired: 2 in, 2 out]
                }
              }
              frame "Start Task 5" {
                n174 = for {
                  shift-right: [w361] -> w356
                  shift-left: w357 -> [w360]
                  tunnel: string[] ["RESET YAW", "RESET ENCODERS", "READ STEPPER VALUES", "Z STEPPER CAM HEIGHT", "", ""] -> [w359] mode=indexing
                  n175 = Enqueue Element(queue=w360, element=w359) -> (queue out=w361:refnum<queue>)  [unwired: 2 in, 2 out]
                }
              }
              frame "Start Task 6" {
                n176 = for {
                  shift-right: [w368] -> w363
                  shift-left: w364 -> [w367]
                  tunnel: string[] ["OPEN LOG CAM ", "", "", "", "", ""] -> [w366] mode=indexing
                  n177 = Enqueue Element(queue=w367, element=w366) -> (queue out=w368:refnum<queue>)  [unwired: 2 in, 2 out]
                }
              }
              frame "None", Default {
              }
              frame "Exit" {
                n178 = for {
                  shift-right: [w377] -> w372
                  shift-left: w373 -> [w376]
                  tunnel: string[] ["STOP", "RESET ENCODERS", "RESET YAW", "EXIT"] -> [w375] mode=indexing
                  n179 = Enqueue Element(queue=w376, element=w375) -> (queue out=w377:refnum<queue>)  [unwired: 2 in, 2 out]
                }
              }
              frame "Start Task 9" {
                n180 = for {
                  shift-right: [w384] -> w380
                  shift-left: w379 -> [w383]
                  tunnel: string[] ["RESET ENCODERS", "READ ENCODERS", "Z STEPPER CAM HEIGHT"] -> [w382] mode=indexing
                  n181 = Enqueue Element(queue=w383, element=w382) -> (queue out=w384:refnum<queue>)  [unwired: 2 in, 2 out]
                }
              }
            }
          }
          frame 5 {
            # ">>> yStepper command>>>"
            n182 = for {
              shift-right: [w393] -> w387
              shift-left: w389 -> [w392]
              tunnel: string[] ["INIT", "RESET ENCODERS", "RESET FLAGS", "CAM CLOSE", "DISPOSE BUFFERS", "EXIT", ""] -> [w391] mode=indexing
              n183 = Enqueue Element(queue=w392, element=w391) -> (queue out=w393:refnum<queue>)  [unwired: 2 in, 2 out]
            }
          }
          frame 6 {
            # ">>> yStepper command>>>"
            # "Use 250"
            n184 = Dequeue Element(queue=w407, timeout in ms (-1)=w406, error in (no error)=w405) -> (element=w404:T7)  [unwired: 3 out]
            n185 = Greater?(x=w398, y=265.0) -> (0:w396:bool)
            n186 = Or(x=w396, y=w399) -> (x .or. y?=w403:bool)
            n187 = case shown="\"None\", Default" w404 {
              tunnel: w403 -> [w410 _]
              tunnel: [w414 State_Type_Definitions."True Stop" ("Enum")] -> w402
              tunnel: w401 -> [w411 w429]
              tunnel: [w409 w428] -> w400
              tunnel: [State_Type_Definitions."Idle" ("Enum") State_Type_Definitions."Shutdown" ("Enum")] -> w395
              frame "None", Default {
                n188 = case shown="True" w410 {
                  tunnel: w411 -> [w417 w423]
                  tunnel: [w416 w421] -> w409
                  frame False {
                    n189 = for {
                      shift-right: [w419] -> w416
                      shift-left: w417 -> [w420]
                      tunnel: string[] ["READ ENCODERS", "READ NAVX", "FORWARD"] ("element") -> [w418] mode=indexing
                      n190 = Enqueue Element(queue=w420, element=w418) -> (queue out=w419:refnum<queue>)  [unwired: 2 in, 2 out]
                    }
                  }
                  frame True {
                    n191 = for {
                      shift-right: [w425] -> w421
                      shift-left: w423 -> [w426]
                      tunnel: string[] ["RESET YAW", "RESET ENCODERS", "STOP", ""] -> [w424] mode=indexing
                      n192 = Enqueue Element(queue=w426, element=w424) -> (queue out=w425:refnum<queue>)  [unwired: 2 in, 2 out]
                    }
                  }
                }
                n193 = Select(t=State_Type_Definitions."True Stop" ("Enum"), s=w410, f=State_Type_Definitions."Task 1" ("Enum")) -> (s? t:f=w414:u16)
              }
              frame "Exit" {
                n194 = for {
                  shift-right: [w433] -> w428
                  shift-left: w429 -> [w434]
                  tunnel: string[] ["STOP", "RESET ENCODERS", "RESET YAW", ""] -> [w432] mode=indexing
                  n195 = Enqueue Element(queue=w434, element=w432) -> (queue out=w433:refnum<queue>)  [unwired: 2 in, 2 out]
                }
              }
            }
          }
          frame 8 {
            # ">> Stepper height reeached >>"
            # ">>> yStepper command>>>"
            # ">> Manual override >>"
            n196 = Dequeue Element(queue=w438, timeout in ms (-1)=w437, error in (no error)=w436) -> (element=w447:T7)  [unwired: 3 out]
            n197 = Equal?(x=w440, y=u8 60) -> (x = y?=w445:bool)
            n198 = case shown="\"None\", Default" w447 {
              tunnel: [w458 State_Type_Definitions."True Stop" ("Enum")] -> w442
              tunnel: [w456 w473] -> w435
              tunnel: w444 -> [w455 _]
              tunnel: w443 -> [w449 _]
              tunnel: [State_Type_Definitions."Idle" ("Enum") State_Type_Definitions."Shutdown" ("Enum")] -> w441
              tunnel: w445 -> [w448 _]
              frame "None", Default {
                # ">> WIill proceed to part ii if not manual override >>"
                # ">>If ENABLE or Trigger is set to true>>"
                n199 = Or(x=w448, y=w449) -> (x .or. y?=w450:bool)
                n200 = case shown="True" w448 {
                  tunnel: [w461 w467] -> w456
                  tunnel: w455 -> [w460 w466]
                  frame False {
                    n201 = for {
                      shift-right: [w463] -> w461
                      shift-left: w460 -> [w464]
                      tunnel: string[] ["Z STEPPER CAM HEIGHT", "READ STEPPER VALUES"] ("element") -> [w462] mode=indexing
                      n202 = Enqueue Element(queue=w464, element=w462) -> (queue out=w463:refnum<queue>)  [unwired: 2 in, 2 out]
                    }
                  }
                  frame True {
                    n203 = for {
                      shift-right: [w469] -> w467
                      shift-left: w466 -> [w470]
                      tunnel: string[] ["ARDUINO - ULTRASONIC", "READ ULTRASONIC", "", "", "", ""] -> [w468] mode=indexing
                      n204 = Enqueue Element(queue=w470, element=w468) -> (queue out=w469:refnum<queue>)  [unwired: 2 in, 2 out]
                    }
                  }
                }
                n205 = Select(t=State_Type_Definitions."True Stop" ("Enum"), s=w449, f=State_Type_Definitions."Task 2:Sensor Mode" ("Enum")) -> (s? t:f=w452:T6)
                n206 = Select(t=w452, s=w450, f=State_Type_Definitions."Task 2:Raise Arm" ("Enum")) -> (s? t:f=w458:T6)
              }
              frame "Exit" {
                n207 = for {
                  shift-right: [w476] -> w473
                  shift-left: _ -> [w477]
                  tunnel: string[] ["STOP", "RESET ENCODERS", "RESET YAW", ""] -> [w475] mode=indexing
                  n208 = Enqueue Element(queue=w477, element=w475) -> (queue out=w476:refnum<queue>)  [unwired: 2 in, 2 out]
                }
              }
            }
          }
          frame 9 {
            w492 = u8 20 ("y")
            # ">>> yStepper command>>>"
            # ">>Object detected>>"
            n209 = Dequeue Element(queue=w484, timeout in ms (-1)=w483, error in (no error)=w482) -> (element=w493:T7)  [unwired: 3 out]
            n210 = Less?(x=w480, y=w492) -> (x < y?=w491:bool)
            n211 = Less?(x=w479, y=w492) -> (x < y?=w490:bool)
            n212 = Or(x=w491, y=w490) -> (x .or. y?=w489:bool)
            "Obstacle detected" <- w489
            n213 = case shown="\"None\", Default" w493 {
              tunnel: w489 -> [w496 _]
              tunnel: [w503 State_Type_Definitions."True Stop" ("Enum")] -> w488
              tunnel: w481 -> [w495 _]
              tunnel: w485 -> [w502 w519]
              tunnel: [w501 w520] -> w487
              tunnel: [State_Type_Definitions."Idle" ("Enum") State_Type_Definitions."Shutdown" ("Enum")] -> w486
              frame "None", Default {
                n214 = case shown="True" w496 {
                  tunnel: w502 -> [w506 w513]
                  tunnel: [w507 w512] -> w501
                  frame False {
                    n215 = for {
                      tunnel: string[] ["READ ULTRASONIC", "STOP"] ("element") -> [w508] mode=indexing
                      shift-right: [w510] -> w507
                      shift-left: w506 -> [w509]
                      n216 = Enqueue Element(queue=w509, element=w508) -> (queue out=w510:refnum<queue>)  [unwired: 2 in, 2 out]
                    }
                  }
                  frame True {
                    n217 = for {
                      shift-right: [w515] -> w512
                      shift-left: w513 -> [w516]
                      tunnel: string[] ["RESET ENCODERS", "READ NAVX", "READ ENCODERS"] -> [w514] mode=indexing
                      n218 = Enqueue Element(queue=w516, element=w514) -> (queue out=w515:refnum<queue>)  [unwired: 2 in, 2 out]
                    }
                  }
                }
                n219 = Or(x=w496, y=w495) -> (x .or. y?=w494:bool)
                n220 = Select(t=State_Type_Definitions."True Stop" ("Enum"), s=w495, f=State_Type_Definitions."Task 2:Reverse Mode" ("Enum")) -> (s? t:f=w497:T6)
                n221 = Select(t=w497, s=w494, f=State_Type_Definitions."Task 2:Sensor Mode" ("Enum")) -> (s? t:f=w503:T6)
              }
              frame "Exit" {
                n222 = for {
                  shift-right: [w523] -> w520
                  shift-left: w519 -> [w524]
                  tunnel: string[] ["STOP", "RESET ENCODERS", "RESET YAW", "ARDUINO MODE 0"] -> [w522] mode=indexing
                  n223 = Enqueue Element(queue=w524, element=w522) -> (queue out=w523:refnum<queue>)  [unwired: 2 in, 2 out]
                }
              }
            }
          }
          frame 10 {
            # ">>> yStepper command>>>"
            n224 = Dequeue Element(queue=w533, timeout in ms (-1)=w534, error in (no error)=w535) -> (element=w537:T7)  [unwired: 3 out]
            n225 = Less?(x=w527, y=-50.0) -> (x < y?=w525:bool)
            n226 = case shown="\"None\", Default" w537 {
              tunnel: [w547 State_Type_Definitions."True Stop" ("Enum")] -> w529
              tunnel: w536 -> [w540 _]
              tunnel: w532 -> [w546 w563]
              tunnel: [w545 w564] -> w528
              tunnel: [State_Type_Definitions."Idle" ("Enum") State_Type_Definitions."Shutdown" ("Enum")] -> w530
              tunnel: w525 -> [w538 _]
              frame "None", Default {
                n227 = case shown="False" w538 {
                  tunnel: w546 -> [w550 w557]
                  tunnel: [w551 w556] -> w545
                  frame False {
                    n228 = for {
                      tunnel: string[] ["READ ENCODERS", "REVERSE", "READ NAVX"] ("element") -> [w552] mode=indexing
                      shift-right: [w554] -> w551
                      shift-left: w550 -> [w553]
                      n229 = Enqueue Element(queue=w553, element=w552) -> (queue out=w554:refnum<queue>)  [unwired: 2 in, 2 out]
                    }
                  }
                  frame True {
                    n230 = for {
                      shift-right: [w559] -> w556
                      shift-left: w557 -> [w560]
                      tunnel: string[] ["STOP", "ARDUINO - ULTRASONIC", "READ ULTRASONIC", "RESET ENCODERS"] -> [w558] mode=indexing
                      n231 = Enqueue Element(queue=w560, element=w558) -> (queue out=w559:refnum<queue>)  [unwired: 2 in, 2 out]
                    }
                  }
                }
                n232 = Or(x=w538, y=w540) -> (x .or. y?=w539:bool)
                n233 = Select(t=State_Type_Definitions."True Stop" ("Enum"), s=w540, f=State_Type_Definitions."Task 2:Sensor Mode" ("Enum")) -> (s? t:f=w541:T6)
                n234 = Select(t=w541, s=w539, f=State_Type_Definitions."Task 2:Reverse Mode" ("Enum")) -> (s? t:f=w547:T6)
              }
              frame "Exit" {
                n235 = for {
                  shift-right: [w567] -> w564
                  shift-left: w563 -> [w568]
                  tunnel: string[] ["STOP", "RESET ENCODERS", "RESET YAW", "ARDUINO MODE 0"] -> [w566] mode=indexing
                  n236 = Enqueue Element(queue=w568, element=w566) -> (queue out=w567:refnum<queue>)  [unwired: 2 in, 2 out]
                }
              }
            }
          }
          frame 11 {
            # ">>> yStepper command>>>"
            n237 = Dequeue Element(queue=w582, timeout in ms (-1)=w581, error in (no error)=w580) -> (element=w571:T7)  [unwired: 3 out]
            n238 = Greater?(x=w579, y=160.0) -> (0:w576:bool)
            n239 = Or(x=w576, y=w577) -> (x .or. y?=w572:bool)
            n240 = case shown="\"None\", Default" w571 {
              tunnel: w572 -> [w585 _]
              tunnel: [w589 State_Type_Definitions."True Stop" ("Enum")] -> w573
              tunnel: w575 -> [w586 w605]
              tunnel: [w584 w604] -> w574
              tunnel: [State_Type_Definitions."Idle" ("Enum") State_Type_Definitions."Shutdown" ("Enum")] -> w570
              frame "None", Default {
                n241 = case shown="False" w585 {
                  tunnel: w586 -> [w592 w598]
                  tunnel: [w591 w596] -> w584
                  frame False {
                    n242 = for {
                      shift-right: [w594] -> w591
                      shift-left: w592 -> [w595]
                      tunnel: string[] ["READ ENCODERS", "R-ACW"] ("element") -> [w593] mode=indexing
                      n243 = Enqueue Element(queue=w595, element=w593) -> (queue out=w594:refnum<queue>)  [unwired: 2 in, 2 out]
                    }
                  }
                  frame True {
                    n244 = for {
                      shift-right: [w600] -> w596
                      shift-left: w598 -> [w601]
                      tunnel: string[] ["RESET YAW", "RESET ENCODERS", "STOP", "ARDUINO MODE 0"] -> [w599] mode=indexing
                      n245 = Enqueue Element(queue=w601, element=w599) -> (queue out=w600:refnum<queue>)  [unwired: 2 in, 2 out]
                    }
                  }
                }
                n246 = Select(t=State_Type_Definitions."True Stop" ("Enum"), s=w585, f=State_Type_Definitions."Task 3" ("Enum")) -> (s? t:f=w589:T6)
              }
              frame "Exit" {
                n247 = for {
                  shift-right: [w608] -> w604
                  shift-left: w605 -> [w609]
                  tunnel: string[] ["STOP", "RESET ENCODERS", "RESET YAW", ""] -> [w607] mode=indexing
                  n248 = Enqueue Element(queue=w609, element=w607) -> (queue out=w608:refnum<queue>)  [unwired: 2 in, 2 out]
                }
              }
            }
          }
          frame 12 {
            # ">> Stepper height reeached >>"
            # ">>> yStepper command>>>"
            # ">> Manual override >>"
            n249 = Dequeue Element(queue=w621, timeout in ms (-1)=w620, error in (no error)=w619) -> (element=w618:T7)  [unwired: 3 out]
            n250 = Equal?(x=w612, y=u8 80) -> (x = y?=w610:bool)
            n251 = case shown="\"Exit\"" w618 {
              tunnel: [w633 State_Type_Definitions."True Stop" ("Enum")] -> w617
              tunnel: [w631 w649] -> w616
              tunnel: w622 -> [w630 w646]
              tunnel: w615 -> [w624 _]
              tunnel: [State_Type_Definitions."Idle" ("Enum") State_Type_Definitions."Shutdown" ("Enum")] -> w614
              tunnel: w610 -> [w623 _]
              frame "None", Default {
                # ">> WIill proceed to part ii if not manual override >>"
                # ">>If ENABLE or Trigger is set to true>>"
                n252 = Or(x=w623, y=w624) -> (x .or. y?=w625:bool)
                n253 = case shown="False" w623 {
                  tunnel: [w636 w642] -> w631
                  tunnel: w630 -> [w635 w641]
                  frame False {
                    n254 = for {
                      shift-right: [w638] -> w636
                      shift-left: w635 -> [w639]
                      tunnel: string[] ["Z STEPPER CAM HEIGHT", "READ STEPPER VALUES"] ("element") -> [w637] mode=indexing
                      n255 = Enqueue Element(queue=w639, element=w637) -> (queue out=w638:refnum<queue>)  [unwired: 2 in, 2 out]
                    }
                  }
                  frame True {
                    n256 = for {
                      shift-right: [w644] -> w642
                      shift-left: w641 -> [w645]
                      tunnel: string[] ["ARDUINO - ULTRASONIC", "READ ULTRASONIC", "FORWARD", "", "", ""] -> [w643] mode=indexing
                      n257 = Enqueue Element(queue=w645, element=w643) -> (queue out=w644:refnum<queue>)  [unwired: 2 in, 2 out]
                    }
                  }
                }
                n258 = Select(t=State_Type_Definitions."True Stop" ("Enum"), s=w624, f=State_Type_Definitions."Task 4_B" ("Enum")) -> (s? t:f=w627:T6)
                n259 = Select(t=w627, s=w625, f=State_Type_Definitions."Task 4_A" ("Enum")) -> (s? t:f=w633:T6)
              }
              frame "Exit" {
                n260 = for {
                  shift-right: [w652] -> w649
                  shift-left: w646 -> [w653]
                  tunnel: string[] ["STOP", "RESET ENCODERS", "RESET YAW", ""] -> [w651] mode=indexing
                  n261 = Enqueue Element(queue=w653, element=w651) -> (queue out=w652:refnum<queue>)  [unwired: 2 in, 2 out]
                }
              }
            }
          }
          frame 13 {
            w657 = u8 20
            # ">> Path blocked >>"
            # ">>> yStepper command>>>"
            # ">> Manual override >>"
            n262 = Dequeue Element(queue=w666, timeout in ms (-1)=w665, error in (no error)=w664) -> (element=w663:T7)  [unwired: 3 out]
            n263 = Less?(x=w659, y=w657) -> (x < y?=w654:bool)
            n264 = Less?(x=w658, y=w657) -> (x < y?=w655:bool)
            n265 = And(x=w655, y=w654) -> (x .and. y?=w656:bool)
            n266 = case shown="\"None\", Default" w663 {
              tunnel: [w680 State_Type_Definitions."True Stop" ("Enum")] -> w668
              tunnel: [w678 w695] -> w669
              tunnel: w662 -> [w677 _]
              tunnel: w667 -> [w671 _]
              tunnel: [State_Type_Definitions."Idle" ("Enum") State_Type_Definitions."Shutdown" ("Enum")] -> w661
              tunnel: w656 -> [w670 _]
              frame "None", Default {
                # ">> Manual override forces program to true stop >>"
                # ">>If ENABLE or Trigger is set to true>>"
                n267 = Or(x=w670, y=w671) -> (x .or. y?=w676:bool)
                n268 = case shown="False" w670 {
                  tunnel: [w683 w688] -> w678
                  tunnel: w677 -> [w682 w687]
                  frame False {
                    n269 = for {
                      shift-right: [w685] -> w683
                      shift-left: w682 -> [w686]
                      tunnel: string[] ["FORWARD", "READ ULTRASONIC", "READ NAVX"] ("element") -> [w684] mode=indexing
                      n270 = Enqueue Element(queue=w686, element=w684) -> (queue out=w685:refnum<queue>)  [unwired: 2 in, 2 out]
                    }
                  }
                  frame True {
                    n271 = for {
                      shift-right: [w691] -> w688
                      shift-left: w687 -> [w692]
                      tunnel: string[] ["STOP", "RESET YAW", "RESET ENCODERS", "RESET FLAGS"] -> [w690] mode=indexing
                      n272 = Enqueue Element(queue=w692, element=w690) -> (queue out=w691:refnum<queue>)  [unwired: 2 in, 2 out]
                    }
                  }
                }
                n273 = Select(t=State_Type_Definitions."True Stop" ("Enum"), s=w671, f=State_Type_Definitions."Task 4_C" ("Enum")) -> (s? t:f=w673:T6)
                n274 = Select(t=w673, s=w676, f=State_Type_Definitions."Task 4_B" ("Enum")) -> (s? t:f=w680:T6)
              }
              frame "Exit" {
                n275 = for {
                  shift-right: [w698] -> w695
                  shift-left: _ -> [w699]
                  tunnel: string[] ["STOP", "RESET ENCODERS", "RESET YAW", ""] -> [w697] mode=indexing
                  n276 = Enqueue Element(queue=w699, element=w697) -> (queue out=w698:refnum<queue>)  [unwired: 2 in, 2 out]
                }
              }
            }
          }
          frame 14 {
            w709 = u8 20
            # ">> xDistance travelled>>"
            # ">> Path NOT blocked >>"
            # ">>> yStepper command>>>"
            # ">> Manual override >>"
            n277 = Dequeue Element(queue=w719, timeout in ms (-1)=w712, error in (no error)=w711) -> (element=w713:T7)  [unwired: 3 out]
            n278 = Greater?(x=w701, y=w709) -> (0:w707:bool)
            n279 = Greater?(x=w706, y=80.0) -> (0:w704:bool)
            n280 = Greater?(x=w700, y=w709) -> (0:w708:bool)
            n281 = And(x=w708, y=w707) -> (x .and. y?=w703:bool)
            n282 = And(x=w704, y=w703) -> (x .and. y?=w702:bool)
            n283 = case shown="\"None\", Default" w713 {
              tunnel: [w730 State_Type_Definitions."True Stop" ("Enum")] -> w716
              tunnel: [w728 w746] -> w715
              tunnel: w718 -> [w727 w743]
              tunnel: w717 -> [w721 _]
              tunnel: [State_Type_Definitions."Idle" ("t") State_Type_Definitions."Shutdown" ("Enum")] -> w714
              tunnel: w702 -> [w720 _]
              frame "None", Default {
                # ">> Manual override forces program to true stop >>"
                # ">>If ENABLE or Trigger is set to true>>"
                n284 = Or(x=w720, y=w721) -> (x .or. y?=w726:bool)
                n285 = case shown="False" w720 {
                  tunnel: [w733 w738] -> w728
                  tunnel: w727 -> [w731 w737]
                  frame False {
                    n286 = for {
                      shift-right: [w735] -> w733
                      shift-left: w731 -> [w736]
                      tunnel: string[] ["RIGHT", "READ NAVX", "READ ENCODERS", "READ ULTRASONIC"] ("element") -> [w734] mode=indexing
                      n287 = Enqueue Element(queue=w736, element=w734) -> (queue out=w735:refnum<queue>)  [unwired: 2 in, 2 out]
                    }
                  }
                  frame True {
                    n288 = for {
                      shift-right: [w741] -> w738
                      shift-left: w737 -> [w742]
                      tunnel: string[] ["STOP", "RESET YAW", "RESET ENCODERS", "ARDUINO - ULTRASONIC"] -> [w740] mode=indexing
                      n289 = Enqueue Element(queue=w742, element=w740) -> (queue out=w741:refnum<queue>)  [unwired: 2 in, 2 out]
                    }
                  }
                }
                n290 = Select(t=State_Type_Definitions."True Stop" ("Enum"), s=w721, f=State_Type_Definitions."Task 4_D" ("Enum")) -> (s? t:f=w722:T6)
                n291 = Select(t=w722, s=w726, f=State_Type_Definitions."Task 4_C" ("Enum")) -> (s? t:f=w730:T6)
              }
              frame "Exit" {
                n292 = for {
                  shift-right: [w749] -> w746
                  shift-left: w743 -> [w750]
                  tunnel: string[] ["STOP", "RESET ENCODERS", "RESET YAW", ""] -> [w748] mode=indexing
                  n293 = Enqueue Element(queue=w750, element=w748) -> (queue out=w749:refnum<queue>)  [unwired: 2 in, 2 out]
                }
              }
            }
          }
          frame 15 {
            w769 = u8 20
            # ">> yDistance travelled>>"
            # ">> Path blocked >>"
            # ">>> yStepper command>>>"
            # ">> Manual override >>"
            n294 = Dequeue Element(queue=w760, timeout in ms (-1)=w759, error in (no error)=w758) -> (element=w770:T7)  [unwired: 3 out]
            n295 = Less?(x=w753, y=w769) -> (x < y?=w767:bool)
            n296 = Greater?(x=w757, y=200.0) -> (0:w765:bool)
            n297 = Less?(x=w752, y=w769) -> (x < y?=w768:bool)
            n298 = And(x=w768, y=w767) -> (x .and. y?=w764:bool)
            n299 = Or(x=w765, y=w764) -> (x .or. y?=w763:bool)
            n300 = case shown="\"None\", Default" w770 {
              tunnel: [w781 State_Type_Definitions."True Stop" ("Enum")] -> w756
              tunnel: [w779 w797] -> w754
              tunnel: w761 -> [w778 w794]
              tunnel: w762 -> [w772 _]
              tunnel: [State_Type_Definitions."Idle" ("t") State_Type_Definitions."Shutdown" ("Enum")] -> w755
              tunnel: w763 -> [w771 _]
              frame "None", Default {
                # ">> Manual override forces program to true stop >>"
                # ">>If ENABLE or Trigger is set to true>>"
                n301 = Or(x=w771, y=w772) -> (x .or. y?=w777:bool)
                n302 = case shown="True" w771 {
                  tunnel: [w784 w789] -> w779
                  tunnel: w778 -> [w782 w788]
                  frame False {
                    n303 = for {
                      shift-right: [w786] -> w784
                      shift-left: w782 -> [w787]
                      tunnel: string[] ["FORWARD", "READ NAVX", "READ ENCODERS", "READ ULTRASONIC"] ("element") -> [w785] mode=indexing
                      n304 = Enqueue Element(queue=w787, element=w785) -> (queue out=w786:refnum<queue>)  [unwired: 2 in, 2 out]
                    }
                  }
                  frame True {
                    n305 = for {
                      shift-right: [w792] -> w789
                      shift-left: w788 -> [w793]
                      tunnel: string[] ["STOP", "RESET YAW", "RESET ENCODERS", "RESET FLAGS"] -> [w791] mode=indexing
                      n306 = Enqueue Element(queue=w793, element=w791) -> (queue out=w792:refnum<queue>)  [unwired: 2 in, 2 out]
                    }
                  }
                }
                n307 = Select(t=State_Type_Definitions."True Stop" ("Enum"), s=w772, f=State_Type_Definitions."True Stop" ("Enum")) -> (s? t:f=w773:T6)
                n308 = Select(t=w773, s=w777, f=State_Type_Definitions."Task 4_D" ("Enum")) -> (s? t:f=w781:T6)
              }
              frame "Exit" {
                n309 = for {
                  shift-right: [w800] -> w797
                  shift-left: w794 -> [w801]
                  tunnel: string[] ["STOP", "RESET ENCODERS", "RESET YAW", ""] -> [w799] mode=indexing
                  n310 = Enqueue Element(queue=w801, element=w799) -> (queue out=w800:refnum<queue>)  [unwired: 2 in, 2 out]
                }
              }
            }
          }
          frame 15 {
            # ">>> yStepper command>>>"
            # ">> Manual override >>"
            n311 = Dequeue Element(queue=w810, timeout in ms (-1)=w809, error in (no error)=w811) -> (element=w808:T7)  [unwired: 3 out]
            n312 = Equal?(x=w807, y=u8 60) -> (x = y?=w805:bool)
            n313 = case shown="\"None\", Default" w808 {
              tunnel: [w821 State_Type_Definitions."True Stop" ("Enum")] -> w812
              tunnel: [w824 w841] -> w813
              tunnel: [State_Type_Definitions."Idle" ("Enum") State_Type_Definitions."Shutdown" ("Enum")] -> w814
              tunnel: w805 -> [w820 _]
              tunnel: w804 -> [w819 _]
              tunnel: w803 -> [w815 w838]
              frame "None", Default {
                # "Stays in Task 5_A until stepper reaches desired \nheight"
                # "T: Go back to idle, F: Continue with task\""
                # ">> Manual override >>"
                n314 = case shown="True" w820 {
                  tunnel: [w828 w834] -> w824
                  tunnel: w815 -> [w826 w832]
                  frame False {
                    n315 = for {
                      tunnel: string[] ["Z STEPPER CAM HEIGHT", "READ STEPPER VALUES"] ("element") -> [w829] mode=indexing
                      shift-right: [w831] -> w828
                      shift-left: w826 -> [w830]
                      n316 = Enqueue Element(queue=w830, element=w829) -> (queue out=w831:refnum<queue>)  [unwired: 2 in, 2 out]
                    }
                  }
                  frame True {
                    n317 = for {
                      shift-right: [w836] -> w834
                      shift-left: w832 -> [w837]
                      tunnel: string[] ["ARDUINO - ULTRASONIC", "READ ULTRASONIC", ""] -> [w835] mode=indexing
                      n318 = Enqueue Element(queue=w837, element=w835) -> (queue out=w836:refnum<queue>)  [unwired: 2 in, 2 out]
                    }
                  }
                }
                n319 = Or(x=w820, y=w819) -> (x .or. y?=w822:bool)
                n320 = Select(t=State_Type_Definitions."True Stop" ("Enum"), s=w819, f=State_Type_Definitions."Task 5B: MOVE TO BOX" ("Enum")) -> (s? t:f=w816:u16)
                n321 = Select(t=w816, s=w822, f=State_Type_Definitions."Task 5A: ARM CAM HEIGHT" ("Enum")) -> (s? t:f=w821:u16)
              }
              frame "Exit" {
                n322 = for {
                  shift-right: [w844] -> w841
                  shift-left: w838 -> [w845]
                  tunnel: string[] ["STOP", "RESET ENCODERS", "RESET YAW", "ARDUINO MODE 0"] -> [w843] mode=indexing
                  n323 = Enqueue Element(queue=w845, element=w843) -> (queue out=w844:refnum<queue>)  [unwired: 2 in, 2 out]
                }
              }
            }
          }
          frame 23 {
            # ">>> yStepper command>>>"
            # ">> Manual override >>"
            n324 = Dequeue Element(queue=w854, timeout in ms (-1)=w853, error in (no error)=w855) -> (element=w852:T7)  [unwired: 3 out]
            n325 = Equal?(x=w851, y=u8 60) -> (x = y?=w849:bool)
            n326 = case shown="\"None\", Default" w852 {
              tunnel: [w865 State_Type_Definitions."True Stop" ("Enum")] -> w856
              tunnel: [w868 w885] -> w857
              tunnel: [State_Type_Definitions."Idle" ("Enum") State_Type_Definitions."Shutdown" ("Enum")] -> w858
              tunnel: w849 -> [w864 _]
              tunnel: w848 -> [w863 _]
              tunnel: w847 -> [w859 w882]
              frame "None", Default {
                # "Stays in Task 5_A until stepper reaches desired \nheight"
                # "T: Go back to idle, F: Continue with task\""
                # ">> Manual override >>"
                n327 = case shown="False" w864 {
                  tunnel: [w872 w878] -> w868
                  tunnel: w859 -> [w870 w876]
                  frame False {
                    n328 = for {
                      tunnel: string[] ["Z STEPPER CAM HEIGHT", "READ STEPPER VALUES"] ("element") -> [w873] mode=indexing
                      shift-right: [w875] -> w872
                      shift-left: w870 -> [w874]
                      n329 = Enqueue Element(queue=w874, element=w873) -> (queue out=w875:refnum<queue>)  [unwired: 2 in, 2 out]
                    }
                  }
                  frame True {
                    n330 = for {
                      shift-right: [w880] -> w878
                      shift-left: w876 -> [w881]
                      tunnel: string[] ["ARDUINO - ULTRASONIC", "READ ULTRASONIC", ""] -> [w879] mode=indexing
                      n331 = Enqueue Element(queue=w881, element=w879) -> (queue out=w880:refnum<queue>)  [unwired: 2 in, 2 out]
                    }
                  }
                }
                n332 = Or(x=w864, y=w863) -> (x .or. y?=w866:bool)
                n333 = Select(t=State_Type_Definitions."True Stop" ("Enum"), s=w863, f=State_Type_Definitions."True Stop" ("Enum")) -> (s? t:f=w860:T6)
                n334 = Select(t=w860, s=w866, f=State_Type_Definitions."Task 5H: RAISE ARM" ("Enum")) -> (s? t:f=w865:T6)
              }
              frame "Exit" {
                n335 = for {
                  shift-right: [w888] -> w885
                  shift-left: w882 -> [w889]
                  tunnel: string[] ["STOP", "RESET ENCODERS", "RESET YAW", "ARDUINO MODE 0"] -> [w887] mode=indexing
                  n336 = Enqueue Element(queue=w889, element=w887) -> (queue out=w888:refnum<queue>)  [unwired: 2 in, 2 out]
                }
              }
            }
          }
          frame 16 {
            w895 = u8 20 ("y")
            # ">>> yStepper command>>>"
            n337 = Less?(x=w892, y=w895) -> (x < y?=w893:bool)
            n338 = Dequeue Element(queue=w899, timeout in ms (-1)=w898, error in (no error)=w900) -> (element=w897:T7)  [unwired: 3 out]
            n339 = Less?(x=w891, y=w895) -> (x < y?=w894:bool)
            n340 = And(x=w894, y=w893) -> (x .and. y?=w890:bool)
            n341 = case shown="\"None\", Default" w897 {
              tunnel: [w912 State_Type_Definitions."True Stop" ("Enum")] -> w902
              tunnel: [w915 w932] -> w901
              tunnel: [State_Type_Definitions."Idle" ("Enum") State_Type_Definitions."Shutdown" ("Enum")] -> w903
              tunnel: w905 -> [w911 _]
              tunnel: w904 -> [w907 w929]
              tunnel: w890 -> [w906 _]
              frame "None", Default {
                # "Stays in Task 5_B to capture image over 5 seconds"
                # "T: Go back to idle, F: Continue with task\""
                # ">> Manual override >>"
                n342 = case shown="True" w906 {
                  tunnel: [w919 w925] -> w915
                  tunnel: w907 -> [w917 w923]
                  frame False {
                    n343 = for {
                      tunnel: string[] ["FORWARD", "READ ULTRASONIC", "READ NAVX"] ("element") -> [w920] mode=indexing
                      shift-right: [w922] -> w919
                      shift-left: w917 -> [w921]
                      n344 = Enqueue Element(queue=w921, element=w920) -> (queue out=w922:refnum<queue>)  [unwired: 2 in, 2 out]
                    }
                  }
                  frame True {
                    n345 = for {
                      shift-right: [w927] -> w925
                      shift-left: w923 -> [w928]
                      tunnel: string[] ["STOP", "RESET ENCODERS", "OPEN LOG CAM", "SET TIMER 5"] -> [w926] mode=indexing
                      n346 = Enqueue Element(queue=w928, element=w926) -> (queue out=w927:refnum<queue>)  [unwired: 2 in, 2 out]
                    }
                  }
                }
                n347 = Or(x=w906, y=w911) -> (x .or. y?=w913:bool)
                n348 = Select(t=State_Type_Definitions."True Stop" ("Enum"), s=w911, f=State_Type_Definitions."Task 5C: CAM BURST" ("Enum")) -> (s? t:f=w908:u16)
                n349 = Select(t=w908, s=w913, f=State_Type_Definitions."Task 5B: MOVE TO BOX" ("Enum")) -> (s? t:f=w912:u16)
              }
              frame "Exit" {
                n350 = for {
                  shift-right: [w935] -> w932
                  shift-left: w929 -> [w936]
                  tunnel: string[] ["STOP", "RESET ENCODERS", "RESET YAW", "ARDUINO MODE 0"] -> [w934] mode=indexing
                  n351 = Enqueue Element(queue=w936, element=w934) -> (queue out=w935:refnum<queue>)  [unwired: 2 in, 2 out]
                }
              }
            }
          }
          frame 17 {
            # ">>> yStepper command>>>"
            # ">> Manual override >>"
            n352 = Dequeue Element(queue=w945, timeout in ms (-1)=w944, error in (no error)=w943) -> (element=w942:T7)  [unwired: 3 out]
            n353 = case shown="\"None\", Default" w942 {
              tunnel: [w954 State_Type_Definitions."True Stop" ("Enum")] -> w947
              tunnel: [w957 w974] -> w940
              tunnel: [State_Type_Definitions."Idle" ("Enum") State_Type_Definitions."Shutdown" ("Enum")] -> w939
              tunnel: w941 -> [w948 _]
              tunnel: w946 -> [w953 w971]
              tunnel: w937 -> [w952 _]
              frame "None", Default {
                # ">> Is time up? >>"
                # "Determines if object is in range to pick up"
                # ">> Manual override >>"
                n354 = case shown="True" w952 {
                  tunnel: [w961 w967] -> w957
                  tunnel: w953 -> [w959 w965]
                  frame False {
                    n355 = for {
                      tunnel: string[] ["CAM ACQ", "START TIMER"] ("element") -> [w962] mode=indexing
                      shift-right: [w964] -> w961
                      shift-left: w959 -> [w963]
                      n356 = Enqueue Element(queue=w963, element=w962) -> (queue out=w964:refnum<queue>)  [unwired: 2 in, 2 out]
                    }
                  }
                  frame True {
                    n357 = for {
                      shift-right: [w969] -> w967
                      shift-left: w965 -> [w970]
                      tunnel: string[] ["CAM CLOSE", "PROCESS IMAGE", "SET TIMER 5"] -> [w968] mode=indexing
                      n358 = Enqueue Element(queue=w970, element=w968) -> (queue out=w969:refnum<queue>)  [unwired: 2 in, 2 out]
                    }
                  }
                }
                n359 = Or(x=w952, y=w948) -> (x .or. y?=w955:bool)
                n360 = Select(t=State_Type_Definitions."True Stop" ("Enum"), s=w948, f=State_Type_Definitions."Task 5D: PROCESS IMAGE" ("Enum")) -> (s? t:f=w950:u16)
                n361 = Select(t=w950, s=w955, f=State_Type_Definitions."Task 5C: CAM BURST" ("Enum")) -> (s? t:f=w954:u16)
              }
              frame "Exit" {
                n362 = for {
                  shift-right: [w977] -> w974
                  shift-left: w971 -> [w978]
                  tunnel: string[] ["STOP", "RESET ENCODERS", "RESET YAW", "ARDUINO MODE 0"] -> [w976] mode=indexing
                  n363 = Enqueue Element(queue=w978, element=w976) -> (queue out=w977:refnum<queue>)  [unwired: 2 in, 2 out]
                }
              }
            }
          }
          frame 18 {
            # ">>> yStepper command>>>"
            n364 = Dequeue Element(queue=w984, timeout in ms (-1)=w983, error in (no error)=w982) -> (element=w981:T7)  [unwired: 3 out]
            n365 = case shown="\"None\", Default" w981 {
              tunnel: [w996 State_Type_Definitions."True Stop" ("Enum")] -> w988
              tunnel: [w999 w1016] -> w987
              tunnel: [State_Type_Definitions."Idle" ("Enum") State_Type_Definitions."Shutdown" ("Enum")] -> w989
              tunnel: w985 -> [w995 _]
              tunnel: w986 -> [w991 w1013]
              tunnel: w979 -> [w990 _]
              frame "None", Default {
                # ">> T: Breaks out of state loop; F: Stays in loop>>"
                # ">> Manual override >>"
                # ">> Checks if time is up>>"
                # "Stays in Task 5D until the object is detected"
                # "T: Go back to idle, F: Continue with task\""
                # ">> Manual override >>"
                n366 = case shown="True" w990 {
                  tunnel: [w1003 w1009] -> w999
                  tunnel: w991 -> [w1001 w1007]
                  frame False {
                    n367 = for {
                      tunnel: string[] ["START TIMER", "PROCESS IMAGE", ""] ("element") -> [w1004] mode=indexing
                      shift-right: [w1006] -> w1003
                      shift-left: w1001 -> [w1005]
                      n368 = Enqueue Element(queue=w1005, element=w1004) -> (queue out=w1006:refnum<queue>)  [unwired: 2 in, 2 out]
                    }
                  }
                  frame True {
                    n369 = for {
                      shift-right: [w1011] -> w1009
                      shift-left: w1007 -> [w1012]
                      tunnel: string[] ["CAM CLOSE", "", ""] -> [w1010] mode=indexing
                      n370 = Enqueue Element(queue=w1012, element=w1010) -> (queue out=w1011:refnum<queue>)  [unwired: 2 in, 2 out]
                    }
                  }
                }
                n371 = Or(x=w990, y=w995) -> (x .or. y?=w997:bool)
                n372 = Select(t=State_Type_Definitions."True Stop" ("Enum"), s=w995, f=State_Type_Definitions."Task 5E: POSITION ARM" ("Enum")) -> (s? t:f=w992:T6)
                n373 = Select(t=w992, s=w997, f=State_Type_Definitions."Task 5D: PROCESS IMAGE" ("Enum")) -> (s? t:f=w996:u16)
              }
              frame "Exit" {
                n374 = for {
                  shift-right: [w1019] -> w1016
                  shift-left: w1013 -> [w1020]
                  tunnel: string[] ["STOP", "RESET ENCODERS", "RESET YAW", "ARDUINO MODE 0"] -> [w1018] mode=indexing
                  n375 = Enqueue Element(queue=w1020, element=w1018) -> (queue out=w1019:refnum<queue>)  [unwired: 2 in, 2 out]
                }
              }
            }
          }
          frame 20 {
            # ">>> yStepper command>>>"
            n376 = Dequeue Element(queue=w1032, timeout in ms (-1)=w1033, error in (no error)=w1034) -> (element=w1036:T7)  [unwired: 3 out]
            n377 = formula code="if (pos < 100)\ny = 42;\n\nelse if (pos >= 100 && pos <= 140)\ny = 30;\n\nelse if (pos >= 141 && pos <= 170)\ny = 25;\n\nelse if (pos >= 171 &&pos <= 180) \ny = 20;\n\nelse if (pos >= 181&& pos <= 200)\ny = 15;\n\nelse if (pos >= 201 && pos <= 230)\ny = 10;\n\nelse if (pos >= 231 && pos <= 320)\ny = 8;\n\nelse if (pos > 320)\ny = 0;"("pos"=w1024) -> ("y"=w1027:dbl)
            n378 = To Unsigned Byte Integer(number=w1027) -> (unsigned 8bit integer=w1022:u8)
            n379 = Equal?(x=w1023, y=w1022) -> (x = y?=w1021:bool)
            n380 = case shown="\"None\", Default" w1036 {
              tunnel: [w1043 State_Type_Definitions."True Stop" ("Enum")] -> w1030
              tunnel: [w1046 w1063] -> w1028
              tunnel: [State_Type_Definitions."Idle" ("Enum") State_Type_Definitions."Shutdown" ("Enum")] -> w1029
              tunnel: w1035 -> [w1042 _]
              tunnel: w1031 -> [w1038 w1060]
              tunnel: w1021 -> [w1037 _]
              frame "None", Default {
                # ">> T: Breaks out of state loop; F: Stays in loop>>"
                # ">> Manual override >>"
                # ">> Checks if time is up>>"
                # "Stays in Task 5D until the object is detected"
                # "T: Go back to idle, F: Continue with task\""
                # ">> Manual override >>"
                n381 = case shown="False" w1037 {
                  tunnel: [w1050 w1056] -> w1046
                  tunnel: w1038 -> [w1048 w1054]
                  frame False {
                    n382 = for {
                      tunnel: string[] ["READ STEPPER VALUES", "Y STEPPER CONTROL", ""] ("element") -> [w1051] mode=indexing
                      shift-right: [w1053] -> w1050
                      shift-left: w1048 -> [w1052]
                      n383 = Enqueue Element(queue=w1052, element=w1051) -> (queue out=w1053:refnum<queue>)  [unwired: 2 in, 2 out]
                    }
                  }
                  frame True {
                    n384 = for {
                      shift-right: [w1058] -> w1056
                      shift-left: w1054 -> [w1059]
                      tunnel: string[] ["CAM CLOSE", "DISPOSE BUFFERS", ""] -> [w1057] mode=indexing
                      n385 = Enqueue Element(queue=w1059, element=w1057) -> (queue out=w1058:refnum<queue>)  [unwired: 2 in, 2 out]
                    }
                  }
                }
                n386 = Or(x=w1037, y=w1042) -> (x .or. y?=w1044:bool)
                n387 = Select(t=State_Type_Definitions."True Stop" ("Enum"), s=w1042, f=State_Type_Definitions."Task 5F: ARM GRAB HEIGHT" ("Enum")) -> (s? t:f=w1039:T6)
                n388 = Select(t=w1039, s=w1044, f=State_Type_Definitions."Task 5E: POSITION ARM" ("Enum")) -> (s? t:f=w1043:T6)
              }
              frame "Exit" {
                n389 = for {
                  shift-right: [w1066] -> w1063
                  shift-left: w1060 -> [w1067]
                  tunnel: string[] ["STOP", "RESET ENCODERS", "RESET YAW", "ARDUINO MODE 0"] -> [w1065] mode=indexing
                  n390 = Enqueue Element(queue=w1067, element=w1065) -> (queue out=w1066:refnum<queue>)  [unwired: 2 in, 2 out]
                }
              }
            }
            n391 = Bundle By Name(cluster=w1026, "yStepper desired"=w1022) -> (w1025:T9)
          }
          frame 21 {
            # ">>> yStepper command>>>"
            # ">> Manual override >>"
            n392 = Dequeue Element(queue=w1076, timeout in ms (-1)=w1075, error in (no error)=w1077) -> (element=w1074:T7)  [unwired: 3 out]
            n393 = Equal?(x=w1073, y=u8 1) -> (x = y?=w1071:bool)
            n394 = case shown="\"None\", Default" w1074 {
              tunnel: [w1087 State_Type_Definitions."True Stop" ("Enum")] -> w1078
              tunnel: [w1090 w1107] -> w1079
              tunnel: [State_Type_Definitions."Idle" ("Enum") State_Type_Definitions."Shutdown" ("Enum")] -> w1080
              tunnel: w1071 -> [w1086 _]
              tunnel: w1070 -> [w1085 _]
              tunnel: w1069 -> [w1081 w1104]
              frame "None", Default {
                # "Stays in Task 5F until stepper reaches desired \nheight"
                # "T: Go back to idle, F: Continue with task\""
                # ">> Manual override >>"
                n395 = case shown="True" w1086 {
                  tunnel: [w1094 w1100] -> w1090
                  tunnel: w1081 -> [w1092 w1098]
                  frame False {
                    n396 = for {
                      tunnel: string[] ["Z STEPPER GRAB HEIGHT", "READ STEPPER VALUES"] ("element") -> [w1095] mode=indexing
                      shift-right: [w1097] -> w1094
                      shift-left: w1092 -> [w1096]
                      n397 = Enqueue Element(queue=w1096, element=w1095) -> (queue out=w1097:refnum<queue>)  [unwired: 2 in, 2 out]
                    }
                  }
                  frame True {
                    n398 = for {
                      shift-right: [w1102] -> w1100
                      shift-left: w1098 -> [w1103]
                      tunnel: string[] ["SET TIMER 5", "CLOSE CLAW", ""] -> [w1101] mode=indexing
                      n399 = Enqueue Element(queue=w1103, element=w1101) -> (queue out=w1102:refnum<queue>)  [unwired: 2 in, 2 out]
                    }
                  }
                }
                n400 = Or(x=w1086, y=w1085) -> (x .or. y?=w1088:bool)
                n401 = Select(t=State_Type_Definitions."True Stop" ("Enum"), s=w1085, f=State_Type_Definitions."Task 5G: CLOSE CLAW" ("Enum")) -> (s? t:f=w1082:T6)
                n402 = Select(t=w1082, s=w1088, f=State_Type_Definitions."Task 5F: ARM GRAB HEIGHT" ("Enum")) -> (s? t:f=w1087:T6)
              }
              frame "Exit" {
                n403 = for {
                  shift-right: [w1110] -> w1107
                  shift-left: w1104 -> [w1111]
                  tunnel: string[] ["STOP", "RESET ENCODERS", "RESET YAW", "ARDUINO MODE 0"] -> [w1109] mode=indexing
                  n404 = Enqueue Element(queue=w1111, element=w1109) -> (queue out=w1110:refnum<queue>)  [unwired: 2 in, 2 out]
                }
              }
            }
          }
          frame 22 {
            # ">>> yStepper command>>>"
            # ">> Manual override >>"
            n405 = Dequeue Element(queue=w1120, timeout in ms (-1)=w1119, error in (no error)=w1118) -> (element=w1117:T7)  [unwired: 3 out]
            n406 = case shown="\"None\", Default" w1117 {
              tunnel: [w1129 State_Type_Definitions."True Stop" ("Enum")] -> w1122
              tunnel: [w1132 w1149] -> w1115
              tunnel: [State_Type_Definitions."Idle" ("Enum") State_Type_Definitions."Shutdown" ("Enum")] -> w1114
              tunnel: w1116 -> [w1123 _]
              tunnel: w1121 -> [w1128 w1146]
              tunnel: w1112 -> [w1127 _]
              frame "None", Default {
                # ">> Is time up? >>"
                # "Determines if object is in range to pick up"
                # ">> Manual override >>"
                n407 = case shown="True" w1127 {
                  tunnel: [w1136 w1142] -> w1132
                  tunnel: w1128 -> [w1134 w1140]
                  frame False {
                    n408 = for {
                      tunnel: string[] ["CLOSE CLAW", "START TIMER"] ("element") -> [w1137] mode=indexing
                      shift-right: [w1139] -> w1136
                      shift-left: w1134 -> [w1138]
                      n409 = Enqueue Element(queue=w1138, element=w1137) -> (queue out=w1139:refnum<queue>)  [unwired: 2 in, 2 out]
                    }
                  }
                  frame True {
                    n410 = for {
                      shift-right: [w1144] -> w1142
                      shift-left: w1140 -> [w1145]
                      tunnel: string[] ["READ STEPPER VALUES", "", ""] -> [w1143] mode=indexing
                      n411 = Enqueue Element(queue=w1145, element=w1143) -> (queue out=w1144:refnum<queue>)  [unwired: 2 in, 2 out]
                    }
                  }
                }
                n412 = Or(x=w1127, y=w1123) -> (x .or. y?=w1130:bool)
                n413 = Select(t=State_Type_Definitions."True Stop" ("Enum"), s=w1123, f=State_Type_Definitions."Task 5H: RAISE ARM" ("Enum")) -> (s? t:f=w1125:T6)
                n414 = Select(t=w1125, s=w1130, f=State_Type_Definitions."Task 5G: CLOSE CLAW" ("Enum")) -> (s? t:f=w1129:T6)
              }
              frame "Exit" {
                n415 = for {
                  shift-right: [w1152] -> w1149
                  shift-left: w1146 -> [w1153]
                  tunnel: string[] ["STOP", "RESET ENCODERS", "RESET YAW", "ARDUINO MODE 0"] -> [w1151] mode=indexing
                  n416 = Enqueue Element(queue=w1153, element=w1151) -> (queue out=w1152:refnum<queue>)  [unwired: 2 in, 2 out]
                }
              }
            }
          }
          frame 24 {
            # ">>> yStepper command>>>"
            n417 = Dequeue Element(queue=w1161, timeout in ms (-1)=w1160, error in (no error)=w1159) -> (element=w1166:T7)  [unwired: 3 out]
            n418 = Equal?(x=w1157, y=u8 60) -> (x = y?=w1156:bool)
            n419 = case shown="\"None\", Default" w1166 {
              tunnel: [w1173 State_Type_Definitions."True Stop" ("Enum")] -> w1164
              tunnel: [w1172 w1190] -> w1163
              tunnel: [State_Type_Definitions."Idle" ("Enum") State_Type_Definitions."Shutdown" ("Enum")] -> w1165
              tunnel: w1162 -> [w1168 _]
              tunnel: w1158 -> [w1170 _]
              tunnel: w1156 -> [w1167 _]
              frame "None", Default {
                n420 = case shown="False" w1167 {
                  tunnel: [w1178 w1184] -> w1172
                  tunnel: w1170 -> [w1176 w1182]
                  frame False {
                    n421 = for {
                      tunnel: string[] ["Z STEPPER CAM HEIGHT", "READ STEPPER VALUES"] ("element") -> [w1179] mode=indexing
                      shift-right: [w1181] -> w1178
                      shift-left: w1176 -> [w1180]
                      n422 = Enqueue Element(queue=w1180, element=w1179) -> (queue out=w1181:refnum<queue>)  [unwired: 2 in, 2 out]
                    }
                  }
                  frame True {
                    n423 = for {
                      shift-right: [w1186] -> w1184
                      shift-left: w1182 -> [w1187]
                      tunnel: string[] ["CAM ACQ", "OPEN LOG CAM"] -> [w1185] mode=indexing
                      n424 = Enqueue Element(queue=w1187, element=w1185) -> (queue out=w1186:refnum<queue>)  [unwired: 2 in, 2 out]
                    }
                  }
                }
                n425 = Or(x=w1167, y=w1168) -> (x .or. y?=w1169:bool)
                n426 = Select(t=State_Type_Definitions."Task 6_B" ("Enum"), s=w1169, f=State_Type_Definitions."Task 6_A" ("Enum")) -> (s? t:f=w1173:T6)
              }
              frame "Exit" {
                n427 = for {
                  shift-right: [w1193] -> w1190
                  shift-left: _ -> [w1194]
                  tunnel: string[] ["STOP", "RESET ENCODERS", "RESET YAW", "ARDUINO MODE 0"] -> [w1192] mode=indexing
                  n428 = Enqueue Element(queue=w1194, element=w1192) -> (queue out=w1193:refnum<queue>)  [unwired: 2 in, 2 out]
                }
              }
            }
          }
          frame 25 {
            # ">>> yStepper command>>>"
            n429 = Dequeue Element(queue=w1204, timeout in ms (-1)=w1202, error in (no error)=w1203) -> (element=w1201:T7)  [unwired: 3 out]
            n430 = case shown="\"None\", Default" w1201 {
              tunnel: [w1211 State_Type_Definitions."True Stop" ("Enum")] -> w1197
              tunnel: [w1210 w1229] -> w1205
              tunnel: [State_Type_Definitions."Idle" ("Enum") State_Type_Definitions."Shutdown" ("Enum")] -> w1198
              tunnel: w1200 -> [w1206 _]
              tunnel: w1199 -> [w1208 _]
              tunnel: w1196 -> [w1207 w1226]
              frame "None", Default {
                # ">> Manual override >>"
                n431 = case shown="True" w1208 {
                  tunnel: [w1216 w1222] -> w1210
                  tunnel: w1207 -> [w1215 w1220]
                  frame False {
                    n432 = for {
                      shift-right: [w1219] -> w1216
                      shift-left: w1215 -> [w1218]
                      tunnel: string[] ["CAM ACQ", "PROCESS IMAGE", "OPEN CLAW"] -> [w1217] mode=indexing
                      n433 = Enqueue Element(queue=w1218, element=w1217) -> (queue out=w1219:refnum<queue>)  [unwired: 2 in, 2 out]
                    }
                  }
                  frame True {
                    n434 = for {
                      shift-right: [w1224] -> w1222
                      shift-left: w1220 -> [w1225]
                      tunnel: string[] ["CAM ACQ", "PROCESS IMAGE", "CLOSE CLAW"] -> [w1223] mode=indexing
                      n435 = Enqueue Element(queue=w1225, element=w1223) -> (queue out=w1224:refnum<queue>)  [unwired: 2 in, 2 out]
                    }
                  }
                }
                n436 = Select(t=State_Type_Definitions."True Stop" ("Enum"), s=w1206, f=State_Type_Definitions."Task 6_B" ("Enum")) -> (s? t:f=w1211:T6)
              }
              frame "Exit" {
                # ">> State after true stop >>"
                # ">> Goes to true stop >>"
                n437 = for {
                  shift-right: [w1232] -> w1229
                  shift-left: w1226 -> [w1233]
                  tunnel: string[] ["STOP", "RESET ENCODERS", "RESET YAW", ""] -> [w1231] mode=indexing
                  n438 = Enqueue Element(queue=w1233, element=w1231) -> (queue out=w1232:refnum<queue>)  [unwired: 2 in, 2 out]
                }
              }
            }
          }
          frame 38 {
            # ">> Stepper height reeached >>"
            # ">>> yStepper command>>>"
            # ">> Manual override >>"
            n439 = Dequeue Element(queue=w1243, timeout in ms (-1)=w1238, error in (no error)=w1242) -> (element=w1246:T7)  [unwired: 3 out]
            n440 = Equal?(x=w1240, y=u8 80) -> (x = y?=w1244:bool)
            n441 = case shown="\"None\", Default" w1246 {
              tunnel: [w1257 State_Type_Definitions."True Stop" ("Enum")] -> w1236
              tunnel: [w1255 w1272] -> w1235
              tunnel: w1239 -> [w1254 _]
              tunnel: w1241 -> [w1248 _]
              tunnel: [State_Type_Definitions."Idle" ("Enum") State_Type_Definitions."Shutdown" ("Enum")] -> w1237
              tunnel: w1244 -> [w1247 _]
              frame "None", Default {
                # ">> WIill proceed to part ii if not manual override >>"
                # ">>If ENABLE or Trigger is set to true>>"
                n442 = Or(x=w1247, y=w1248) -> (x .or. y?=w1249:bool)
                n443 = case shown="True" w1247 {
                  tunnel: [w1260 w1266] -> w1255
                  tunnel: w1254 -> [w1259 w1265]
                  frame False {
                    n444 = for {
                      shift-right: [w1262] -> w1260
                      shift-left: w1259 -> [w1263]
                      tunnel: string[] ["Z STEPPER CAM HEIGHT", "READ STEPPER VALUES"] ("element") -> [w1261] mode=indexing
                      n445 = Enqueue Element(queue=w1263, element=w1261) -> (queue out=w1262:refnum<queue>)  [unwired: 2 in, 2 out]
                    }
                  }
                  frame True {
                    n446 = for {
                      shift-right: [w1268] -> w1266
                      shift-left: w1265 -> [w1269]
                      tunnel: string[] ["ARDUINO - ULTRASONIC", "READ ULTRASONIC", "", "", "", ""] -> [w1267] mode=indexing
                      n447 = Enqueue Element(queue=w1269, element=w1267) -> (queue out=w1268:refnum<queue>)  [unwired: 2 in, 2 out]
                    }
                  }
                }
                n448 = Select(t=State_Type_Definitions."True Stop" ("Enum"), s=w1248, f=State_Type_Definitions."Task 9B: Rotate to Angle" ("Enum")) -> (s? t:f=w1251:T6)
                n449 = Select(t=w1251, s=w1249, f=State_Type_Definitions."Task 9A: Raise Arm" ("Enum")) -> (s? t:f=w1257:T6)
              }
              frame "Exit" {
                n450 = for {
                  shift-right: [w1275] -> w1272
                  shift-left: _ -> [w1276]
                  tunnel: string[] ["STOP", "RESET ENCODERS", "RESET YAW", ""] -> [w1274] mode=indexing
                  n451 = Enqueue Element(queue=w1276, element=w1274) -> (queue out=w1275:refnum<queue>)  [unwired: 2 in, 2 out]
                }
              }
            }
          }
          frame 39 {
            # ">>> yStepper command>>>"
            n452 = Dequeue Element(queue=w1288, timeout in ms (-1)=w1287, error in (no error)=w1286) -> (element=w1290:T7)  [unwired: 3 out]
            n453 = In Range and Coerce(upper limit=305.0, x=w1280, lower limit=295.0) -> (In Range?=w1277:bool)  [unwired: 1 out]
            n454 = case shown="\"None\", Default" w1290 {
              tunnel: w1281 -> [w1293 _]
              tunnel: [w1301 State_Type_Definitions."True Stop" ("Enum")] -> w1283
              tunnel: w1289 -> [w1299 w1317]
              tunnel: [w1298 w1316] -> w1282
              tunnel: [State_Type_Definitions."Idle" ("Enum") State_Type_Definitions."Shutdown" ("Enum")] -> w1284
              tunnel: w1277 -> [w1291 _]
              frame "None", Default {
                n455 = Or(x=w1291, y=w1293) -> (x .or. y?=w1292:bool)
                n456 = case shown="True" w1291 {
                  tunnel: w1299 -> [w1304 w1310]
                  tunnel: [w1303 w1308] -> w1298
                  frame False {
                    n457 = for {
                      shift-right: [w1306] -> w1303
                      shift-left: w1304 -> [w1307]
                      tunnel: string[] ["READ NAVX", "R-ACW"] ("element") -> [w1305] mode=indexing
                      n458 = Enqueue Element(queue=w1307, element=w1305) -> (queue out=w1306:refnum<queue>)  [unwired: 2 in, 2 out]
                    }
                  }
                  frame True {
                    n459 = for {
                      shift-right: [w1312] -> w1308
                      shift-left: w1310 -> [w1313]
                      tunnel: string[] ["STOP", "RESET ENCODERS", "RESET YAW", ""] -> [w1311] mode=indexing
                      n460 = Enqueue Element(queue=w1313, element=w1311) -> (queue out=w1312:refnum<queue>)  [unwired: 2 in, 2 out]
                    }
                  }
                }
                n461 = Select(t=State_Type_Definitions."True Stop" ("Enum"), s=w1293, f=State_Type_Definitions."Task 9C: Rotation alignmnet") -> (s? t:f=w1295:u16)
                n462 = Select(t=w1295, s=w1292, f=State_Type_Definitions."Task 9B: Rotate to Angle" ("Enum")) -> (s? t:f=w1301:u16)
              }
              frame "Exit" {
                n463 = for {
                  shift-right: [w1320] -> w1316
                  shift-left: w1317 -> [w1321]
                  tunnel: string[] ["STOP", "RESET ENCODERS", "RESET YAW", ""] -> [w1319] mode=indexing
                  n464 = Enqueue Element(queue=w1321, element=w1319) -> (queue out=w1320:refnum<queue>)  [unwired: 2 in, 2 out]
                }
              }
            }
          }
          frame 33 {
            # ">>> yStepper command>>>"
            n465 = Dequeue Element(queue=w1330, timeout in ms (-1)=w1329, error in (no error)=w1328) -> (element=w1331:T7)  [unwired: 3 out]
            n466 = case shown="\"None\", Default" w1331 {
              tunnel: w1326 -> [w1332 _]
              tunnel: [w1340 State_Type_Definitions."True Stop" ("Enum")] -> w1323
              tunnel: w1327 -> [w1338 w1356]
              tunnel: [w1337 w1355] -> w1322
              tunnel: [State_Type_Definitions."Idle" ("Enum") State_Type_Definitions."Shutdown" ("Enum")] -> w1325
              frame "None", Default {
                n467 = case shown="True" w1332 {
                  tunnel: w1338 -> [w1343 w1349]
                  tunnel: [w1342 w1347] -> w1337
                  frame False {
                    n468 = for {
                      shift-right: [w1345] -> w1342
                      shift-left: w1343 -> [w1346]
                      tunnel: string[] ["READ IR", "FORWARD - IR ASSIST"] ("element") -> [w1344] mode=indexing
                      n469 = Enqueue Element(queue=w1346, element=w1344) -> (queue out=w1345:refnum<queue>)  [unwired: 2 in, 2 out]
                    }
                  }
                  frame True {
                    n470 = for {
                      shift-right: [w1351] -> w1347
                      shift-left: w1349 -> [w1352]
                      tunnel: string[] ["STOP", "RESET ENCODERS", "RESET YAW", ""] -> [w1350] mode=indexing
                      n471 = Enqueue Element(queue=w1352, element=w1350) -> (queue out=w1351:refnum<queue>)  [unwired: 2 in, 2 out]
                    }
                  }
                }
                n472 = Select(t=State_Type_Definitions."True Stop" ("Enum"), s=w1332, f=State_Type_Definitions."True Stop") -> (s? t:f=w1334:T6)
                n473 = Select(t=w1334, s=w1332, f=State_Type_Definitions."Task 9C: Rotation alignmnet" ("Enum")) -> (s? t:f=w1340:u16)
              }
              frame "Exit" {
                n474 = for {
                  shift-right: [w1359] -> w1355
                  shift-left: w1356 -> [w1360]
                  tunnel: string[] ["STOP", "RESET ENCODERS", "RESET YAW", ""] -> [w1358] mode=indexing
                  n475 = Enqueue Element(queue=w1360, element=w1358) -> (queue out=w1359:refnum<queue>)  [unwired: 2 in, 2 out]
                }
              }
            }
          }
        }
      }
    }
    n476 = local write "Green LED"(w197) -> ()
  }
  n477 = call <vilib>:"DIO Close.vi"("error in (no error)"=w23, "DIO Info In"=w26) -> ()  [unwired: 9 in, 1 out]
  n478 = call <vilib>:"DIO Close.vi"("error in (no error)"=w33, "DIO Info In"=w35) -> ()  [unwired: 9 in, 1 out]
  n479 = call <vilib>:"NavX Close.vi"("error in (no error)"=w7, "NavX Info In"=w6) -> ()  [unwired: 9 in, 1 out]
  n480 = call <vilib>:"DIO Close.vi"("error in (no error)"=w28, "DIO Info In"=w30) -> ()  [unwired: 9 in, 1 out]
  n481 = call <vilib>:"DIO Close.vi"("error in (no error)"=w14, "DIO Info In"=w15) -> ()  [unwired: 9 in, 1 out]
  n482 = call <vilib>:"DIO Close.vi"("error in (no error)"=w9, "DIO Info In"=w10) -> ()  [unwired: 9 in, 1 out]
  n483 = while {
    stop <- w1908 stop-if-true
    n484 = call <vilib>:"RT Get CPU Loads.vi"() -> ("CPU loads"=→"CPU loads":T5[])  [unwired: 10 in, 1 out]
    n485 = Wait (ms)(milliseconds to wait=u32 100) -> ()  [unwired: 1 out]
    n486 = call "FGV Bool.vi"("Init/Read/Write State"=States_for_Action_Engine."Read") -> ("Output node"=w1908:bool)  [unwired: 2 in, 1 out]
  }
  n487 = while {
    stop <- w1912 stop-if-true
    n488 = call "MOTOR CONTROL WITH PID AE.vi"("AE Mode"=MOTOR_CONTROL_WITH_PID_AE_DATA_MODE_TYPE_DEF."Read from AE") -> ("Speed & distance"=→"Speed & distance":T1)  [unwired: 3 in]
    n489 = call "FGV Bool.vi"("Init/Read/Write State"=States_for_Action_Engine."Read") -> ("Output node"=w1912:bool)  [unwired: 2 in, 1 out]
    n490 = Wait (ms)(milliseconds to wait=u32 5) -> ()  [unwired: 1 out]
  }
  n491 = Merge Errors "Merge Errors"(w63, w62) -> (w45:errorcluster)
  n492 = Merge Errors(w49, w45) -> (w44:errorcluster)
  n493 = Destroy User Event(user event=w66, error in=w44) -> ()  [unwired: 1 out]
  n494 = Destroy User Event(user event=w67, error in=w44) -> ()  [unwired: 1 out]
  n495 = Unregister For Events(event registration refnum=w58, error in=w44) -> ()  [unwired: 1 out]
  n496 = Release Queue(queue=w40, error in (no error)=w44) -> (error out=→"error out":errorcluster)  [unwired: 1 in, 2 out]
  n497 = Release Queue(queue=w57, error in (no error)=w44) -> ()  [unwired: 1 in, 3 out]
